vi "HitrapGUI.HTLE_TR6BT1.vi"() -> ()   [LabVIEW 2014, in "HitrapGUI.lvlib"]
uses:
  HitrapGUI.lvlib
  CSlibraries/GUILib/GUILib.userEventsMainType.ctl
  CSlibraries-extern/DimLVEvent/DimIndicators/DimIndicators.anyType.ctl
  CSlibraries/GUILib/GUILib.simpleNumeric.ctl
  CSlibraries/GUILib/GUILib.basicNumeric.ctl
  CSlibraries/UtilityLib/UtilityLib.valueStatus.ctl
  CSCore/CSSystem/CoreDefs/CoreDefs.rawDataType.ctl
  CSCore/CSSystem/CoreLib/CoreLib.double 2 byte array.vi
  CSlibraries/UtilityLib/UtilityLib.lvlib
  CSCore/CSSystem/CSSystemLib/CSSystemLib.lvlib
  CSlibraries-extern/DimLVEvent/DimIndicators/DimIndicators.lvlib
  CSCore/GUIs/GOGControllerGUI/GOGControllerGUI.lvlib
  CSlibraries/GUILib/GUILib.lvlib
  CSCore/CSSystem/CoreLib/CoreLib.lvlib
panel:
  in  "userEventsMain 2":T1
  in  "userEventsMain":T1
  in  "Next":bool
  in  "Previous":bool
  in  "APS_ch1":bool=TRUE
  in  "APS_ch1Ctl":T2 {"nom" step=1.0}
  in  "APS_ch2Ctl":T2 {"nom" step=1.0}
  in  "APS_ch2":bool=TRUE
  in  "All Low   All High":bool
  in  "High21":bool
  in  "High20":bool
  in  "High19":bool
  in  "High18":bool
  in  "High17":bool
  in  "High15":bool
  in  "High16":bool
  in  "High13":bool
  in  "High14":bool
  in  "High11":bool
  in  "High12":bool
  in  "High9":bool
  in  "High10":bool
  in  "High5":bool
  in  "High6":bool
  in  "High7":bool
  in  "High8":bool
  in  "High4":bool
  in  "High3":bool
  in  "High2":bool
  in  "High1":bool
  out "XY Graph":cluster{dbl, "Value":dbl}[](graph)
  in  "TR6BT1 SetModeCtl":T2 caption="TR6BT1Trap1Ctl" {"nom" step=1.0}
  in  "TR6BT1 SetMode":bool=TRUE
  in  "Enum":enum16{"Voltage1", "Voltage2"}(ring)
  in  "LowVoltage      HighVoltage":bool
  in  "TR6BT1Trap11Ctl":cluster{"nom":T3, "act":dbl, "inc":dbl} {"nom" step=1.0}
  in  "TR6BT1Trap10Ctl":cluster{"nom":T3, "act":dbl, "inc":dbl} {"nom" step=1.0}
  in  "TR6BT1Trap9Ctl":cluster{"nom":T3, "act":dbl, "inc":dbl} {"nom" step=1.0}
  in  "TR6BT1Trap7Ctl":cluster{"nom":T3, "act":dbl, "inc":dbl} {"nom" step=1.0}
  in  "TR6BT1Trap5Ctl":cluster{"nom":T3, "act":dbl, "inc":dbl} {"nom" step=1.0}
  in  "TR6BT1Trap12Ctl":cluster{"nom":T3, "act":dbl, "inc":dbl} {"nom" step=1.0}
  in  "TR6BT1Trap21Ctl":cluster{"nom":T3, "act":dbl, "inc":dbl} {"nom" step=1.0}
  in  "TR6BT1Trap8Ctl":cluster{"nom":T3, "act":dbl, "inc":dbl} {"nom" step=1.0}
  in  "TR6BT1Trap6Ctl":cluster{"nom":T3, "act":dbl, "inc":dbl} {"nom" step=1.0}
  in  "TR6BT1Trap4Ctl":cluster{"nom":T3, "act":dbl, "inc":dbl} {"nom" step=1.0}
  in  "TR6BT1Trap2Ctl":cluster{"nom":T3, "act":dbl, "inc":dbl} {"nom" step=1.0}
  in  "TR6BT1Trap3Ctl":cluster{"nom":T3, "act":dbl, "inc":dbl} {"nom" step=1.0}
  in  "TR6BT1Trap19Ctl":cluster{"nom":T3, "act":dbl, "inc":dbl} {"nom" step=1.0}
  in  "TR6BT1Trap20Ctl":cluster{"nom":T3, "act":dbl, "inc":dbl} {"nom" step=1.0}
  in  "TR6BT1Trap18Ctl":cluster{"nom":T3, "act":dbl, "inc":dbl} {"nom" step=1.0}
  in  "TR6BT1Trap17Ctl":cluster{"nom":T3, "act":dbl, "inc":dbl} {"nom" step=1.0}
  in  "TR6BT1Trap16Ctl":cluster{"nom":T3, "act":dbl, "inc":dbl} {"nom" step=1.0}
  in  "TR6BT1Trap15Ctl":cluster{"nom":T3, "act":dbl, "inc":dbl} {"nom" step=1.0}
  in  "TR6BT1Trap14Ctl":cluster{"nom":T3, "act":dbl, "inc":dbl} {"nom" step=1.0}
  in  "TR6BT1Trap13Ctl":cluster{"nom":T3, "act":dbl, "inc":dbl} {"nom" step=1.0}
  in  "TR6BT1Trap1Ctl":cluster{"nom":T3, "act":dbl, "inc":dbl} {"nom" step=1.0}
  in  "TR6BT1Trap11_HCtl":cluster{"nom":T3, "act":dbl, "inc":dbl} {"nom" step=1.0}
  in  "TR6BT1Trap10_HCtl":cluster{"nom":T3, "act":dbl, "inc":dbl} {"nom" step=1.0}
  in  "TR6BT1Trap4_HCtl":cluster{"nom":T3, "act":dbl, "inc":dbl} {"nom" step=1.0}
  in  "TR6BT1Trap9_HCtl":cluster{"nom":T3, "act":dbl, "inc":dbl} {"nom" step=1.0}
  in  "TR6BT1Trap12_HCtl":cluster{"nom":T3, "act":dbl, "inc":dbl} {"nom" step=1.0}
  in  "TR6BT1Trap21_HCtl":cluster{"nom":T3, "act":dbl, "inc":dbl} {"nom" step=1.0}
  in  "TR6BT1Trap8_HCtl":cluster{"nom":T3, "act":dbl, "inc":dbl} {"nom" step=1.0}
  in  "TR6BT1Trap7_HCtl":cluster{"nom":T3, "act":dbl, "inc":dbl} {"nom" step=1.0}
  in  "TR6BT1Trap6_HCtl":cluster{"nom":T3, "act":dbl, "inc":dbl} {"nom" step=1.0}
  in  "TR6BT1Trap5_HCtl":cluster{"nom":T3, "act":dbl, "inc":dbl} {"nom" step=1.0}
  in  "TR6BT1Trap3_HCtl":cluster{"nom":T3, "act":dbl, "inc":dbl} {"nom" step=1.0}
  in  "TR6BT1Trap2_HCtl":cluster{"nom":T3, "act":dbl, "inc":dbl} {"nom" step=1.0}
  in  "TR6BT1Trap20_HCtl":cluster{"nom":T3, "act":dbl, "inc":dbl} {"nom" step=1.0}
  in  "TR6BT1Trap17_HCtl":cluster{"nom":T3, "act":dbl, "inc":dbl} {"nom" step=1.0}
  in  "TR6BT1Trap18_HCtl":cluster{"nom":T3, "act":dbl, "inc":dbl} {"nom" step=1.0}
  in  "TR6BT1Trap19_HCtl":cluster{"nom":T3, "act":dbl, "inc":dbl} {"nom" step=1.0}
  in  "TR6BT1Trap16_HCtl":cluster{"nom":T3, "act":dbl, "inc":dbl} {"nom" step=1.0}
  in  "TR6BT1Trap15_HCtl":cluster{"nom":T3, "act":dbl, "inc":dbl} {"nom" step=1.0}
  in  "TR6BT1Trap14_HCtl":cluster{"nom":T3, "act":dbl, "inc":dbl} {"nom" step=1.0}
  in  "TR6BT1Trap13_HCtl":cluster{"nom":T3, "act":dbl, "inc":dbl} {"nom" step=1.0}
  in  "TR6BT1Trap1_HCtl":cluster{"nom":T3, "act":dbl, "inc":dbl} {"nom" step=1.0}
  in  "TR6BT1Trap2":bool=TRUE
  in  "TR6BT1Trap21":bool=TRUE
  in  "TR6BT1Trap20":bool=TRUE
  in  "TR6BT1Trap19":bool=TRUE
  in  "TR6BT1Trap18":bool=TRUE
  in  "TR6BT1Trap17":bool=TRUE
  in  "TR6BT1Trap16":bool=TRUE
  in  "TR6BT1Trap15":bool=TRUE
  in  "TR6BT1Trap14":bool=TRUE
  in  "TR6BT1Trap13":bool=TRUE
  in  "TR6BT1Trap12":bool=TRUE
  in  "TR6BT1Trap11":bool=TRUE
  in  "TR6BT1Trap10":bool=TRUE
  in  "TR6BT1Trap9":bool=TRUE
  in  "TR6BT1Trap8":bool=TRUE
  in  "TR6BT1Trap7":bool=TRUE
  in  "TR6BT1Trap6":bool=TRUE
  in  "TR6BT1Trap5":bool=TRUE
  in  "TR6BT1Trap4":bool=TRUE
  in  "TR6BT1Trap3":bool=TRUE
  in  "TR6BT1Trap1":bool=TRUE
  in  "TR6BT1Trap12/2":bool=TRUE
  in  "TR6BT1Trap11/8":bool=TRUE
  in  "TR6BT1Trap11/7":bool=TRUE
  in  "TR6BT1Trap11/6":bool=TRUE
  in  "TR6BT1Trap11/5":bool=TRUE
  in  "TR6BT1Trap11/4":bool=TRUE
  in  "TR6BT1Trap11/3":bool=TRUE
  in  "TR6BT1Trap11/2":bool=TRUE
  in  "TR6BT1Trap10/2":bool=TRUE
  in  "TR6BT1Trap12/2_H":bool=TRUE
  in  "TR6BT1Trap11/8_H":bool=TRUE
  in  "TR6BT1Trap11/7_H":bool=TRUE
  in  "TR6BT1Trap11/6_H":bool=TRUE
  in  "TR6BT1Trap11/5_H":bool=TRUE
  in  "TR6BT1Trap11/4_H":bool=TRUE
  in  "TR6BT1Trap11/3_H":bool=TRUE
  in  "TR6BT1Trap11/2_H":bool=TRUE
  in  "TR6BT1Trap10/2_H":bool=TRUE
  in  "TR6BT1Trap12/2Ctl":T2 {"nom" step=1.0}
  in  "TR6BT1Trap11/8Ctl":T2 {"nom" step=1.0}
  in  "TR6BT1Trap11/7Ctl":T2 {"nom" step=1.0}
  in  "TR6BT1Trap11/6Ctl":T2 {"nom" step=1.0}
  in  "TR6BT1Trap11/5Ctl":T2 {"nom" step=1.0}
  in  "TR6BT1Trap11/4Ctl":T2 {"nom" step=1.0}
  in  "TR6BT1Trap11/3Ctl":T2 {"nom" step=1.0}
  in  "TR6BT1Trap11/2Ctl":T2 {"nom" step=1.0}
  in  "TR6BT1Trap10/2Ctl":T2 {"nom" step=1.0}
  in  "TR6BT1Trap12/2_HCtl":T2 {"nom" step=1.0}
  in  "TR6BT1Trap11/8_HCtl":T2 {"nom" step=1.0}
  in  "TR6BT1Trap11/7_HCtl":T2 {"nom" step=1.0}
  in  "TR6BT1Trap11/6_HCtl":T2 {"nom" step=1.0}
  in  "TR6BT1Trap11/5_HCtl":T2 {"nom" step=1.0}
  in  "TR6BT1Trap11/4_HCtl":T2 {"nom" step=1.0}
  in  "TR6BT1Trap11/3_HCtl":T2 {"nom" step=1.0}
  in  "TR6BT1Trap11/2_HCtl":T2 {"nom" step=1.0}
  in  "TR6BT1Trap10/2_HCtl":T2 {"nom" step=1.0}
  in  "TR6BT1Trap17_H":bool=TRUE
  in  "TR6BT1Trap16_H":bool=TRUE
  in  "TR6BT1Trap15_H":bool=TRUE
  in  "TR6BT1Trap14_H":bool=TRUE
  in  "TR6BT1Trap13_H":bool=TRUE
  in  "TR6BT1Trap12_H":bool=TRUE
  in  "TR6BT1Trap8_H":bool=TRUE
  in  "TR6BT1Trap7_H":bool=TRUE
  in  "TR6BT1Trap5_H":bool=TRUE
  in  "TR6BT1Trap4_H":bool=TRUE
  in  "TR6BT1Trap3_H":bool=TRUE
  in  "TR6BT1Trap2_H":bool=TRUE
  in  "TR6BT1Trap21_H":bool=TRUE
  in  "TR6BT1Trap20_H":bool=TRUE
  in  "TR6BT1Trap19_H":bool=TRUE
  in  "TR6BT1Trap18_H":bool=TRUE
  in  "TR6BT1Trap11_H":bool=TRUE
  in  "TR6BT1Trap10_H":bool=TRUE
  in  "TR6BT1Trap9_H":bool=TRUE
  in  "TR6BT1Trap6_H":bool=TRUE
  in  "TR6BT1Trap1_H":bool=TRUE
  in  "OK Button":bool
  in  "analog1Ctl":T2 {"nom" step=1.0}
  in  "analog1":bool=TRUE
  out "subSystem1State":string
  in  "subSystem1":bool
  out "subSystem1StateQuality":string
  in  "subControllersIgnoredDIM":T4
  in  "iniData":string
  in  "stop":bool
  in  "dummy":bool
  in  "parentSystem":bool
  in  "userEvent":refnum<user-event>
  # "TR6BT1"
  # "Amplifier"
  # "1"
  # "2"
  # "3"
  # "4"
  # "5"
  # "6"
  # "7"
  # "8"
  # "9"
  # "10"
  # "11"
  # "12"
  # "13"
  # "14"
  # "15"
  # "16"
  # "17"
  # "18"
  # "19"
  # "20"
  # "21"
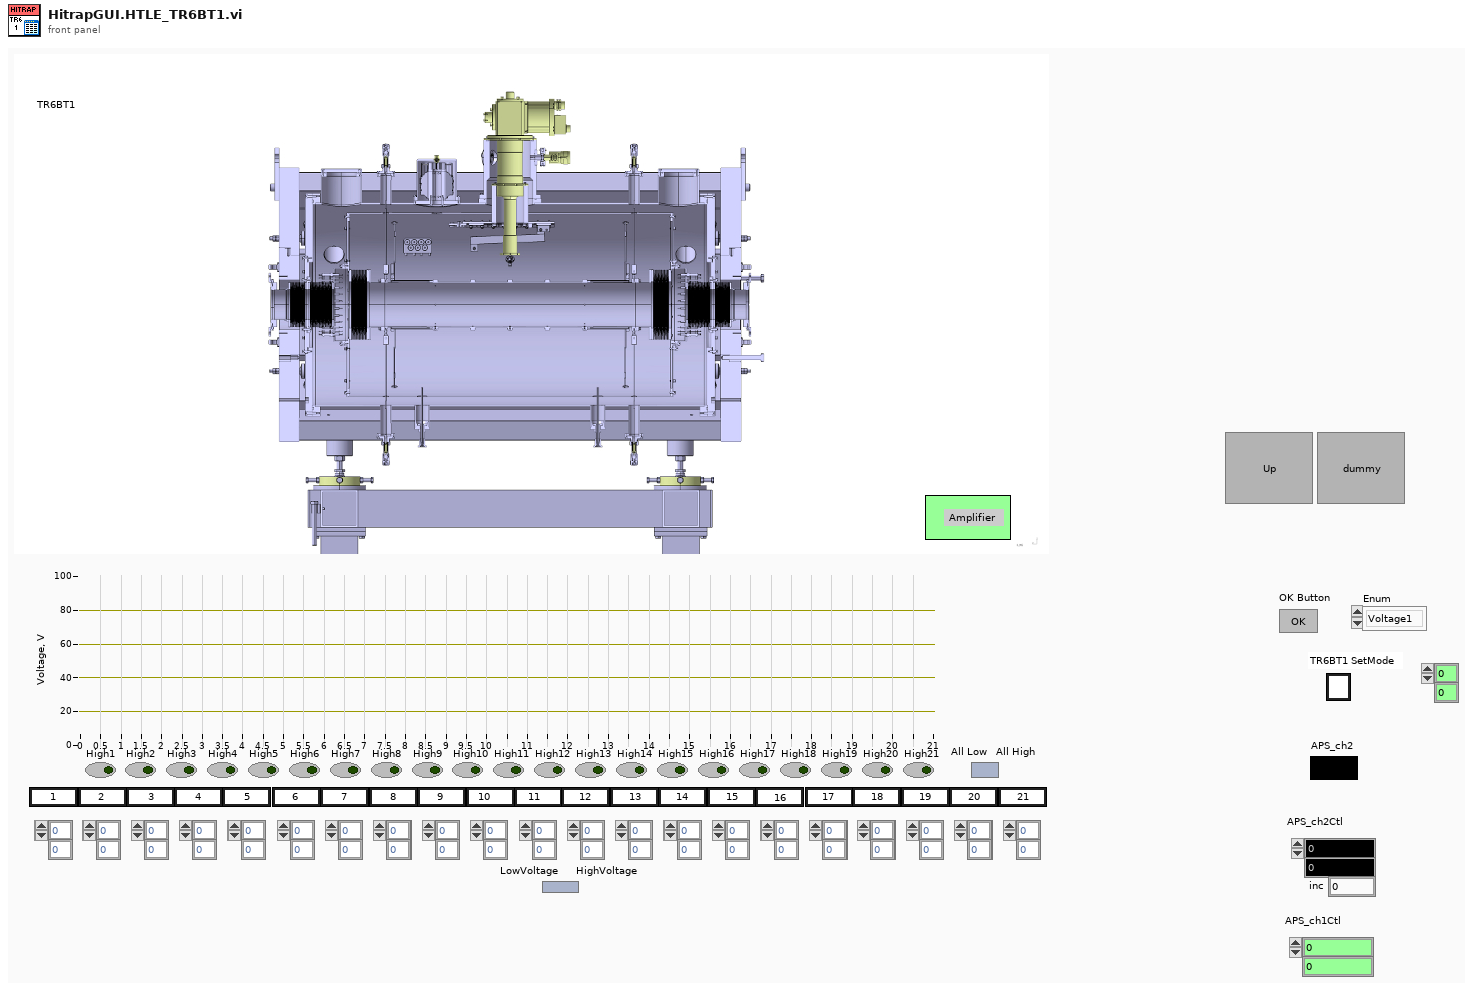
[diagram p1: front panel]
types:
  T1 = typedef "GUILib.lvlib/GUILib.userEventsMainType.ctl" = cluster{"data":string, "dataType":i32}
  T2 = typedef "GUILib.lvlib/GUILib.simpleNumeric.ctl" = cluster{"nom":T3, "act":dbl, "inc":dbl}
  T3 = typedef "GUILib.lvlib/GUILib.basicNumeric.ctl" = dbl
  T4 = typedef "DimIndicators.lvlib/DimIndicators.anyType.ctl" = cluster{"data":string, "no link":bool, "quality":i32, "timeStamp":dbl}
  T5 = typedef "UtilityLib.lvlib/UtilityLib.valueStatus.ctl" = enum16{"no info available", "stand by/off", "on", "warning", "alarm/malfunction", "not implemented", "user action required", "important information", "system default", "control default", "indicator default", "button default"}
  T6 = typedef "CoreDefs.rawDataType.ctl" = i8[]
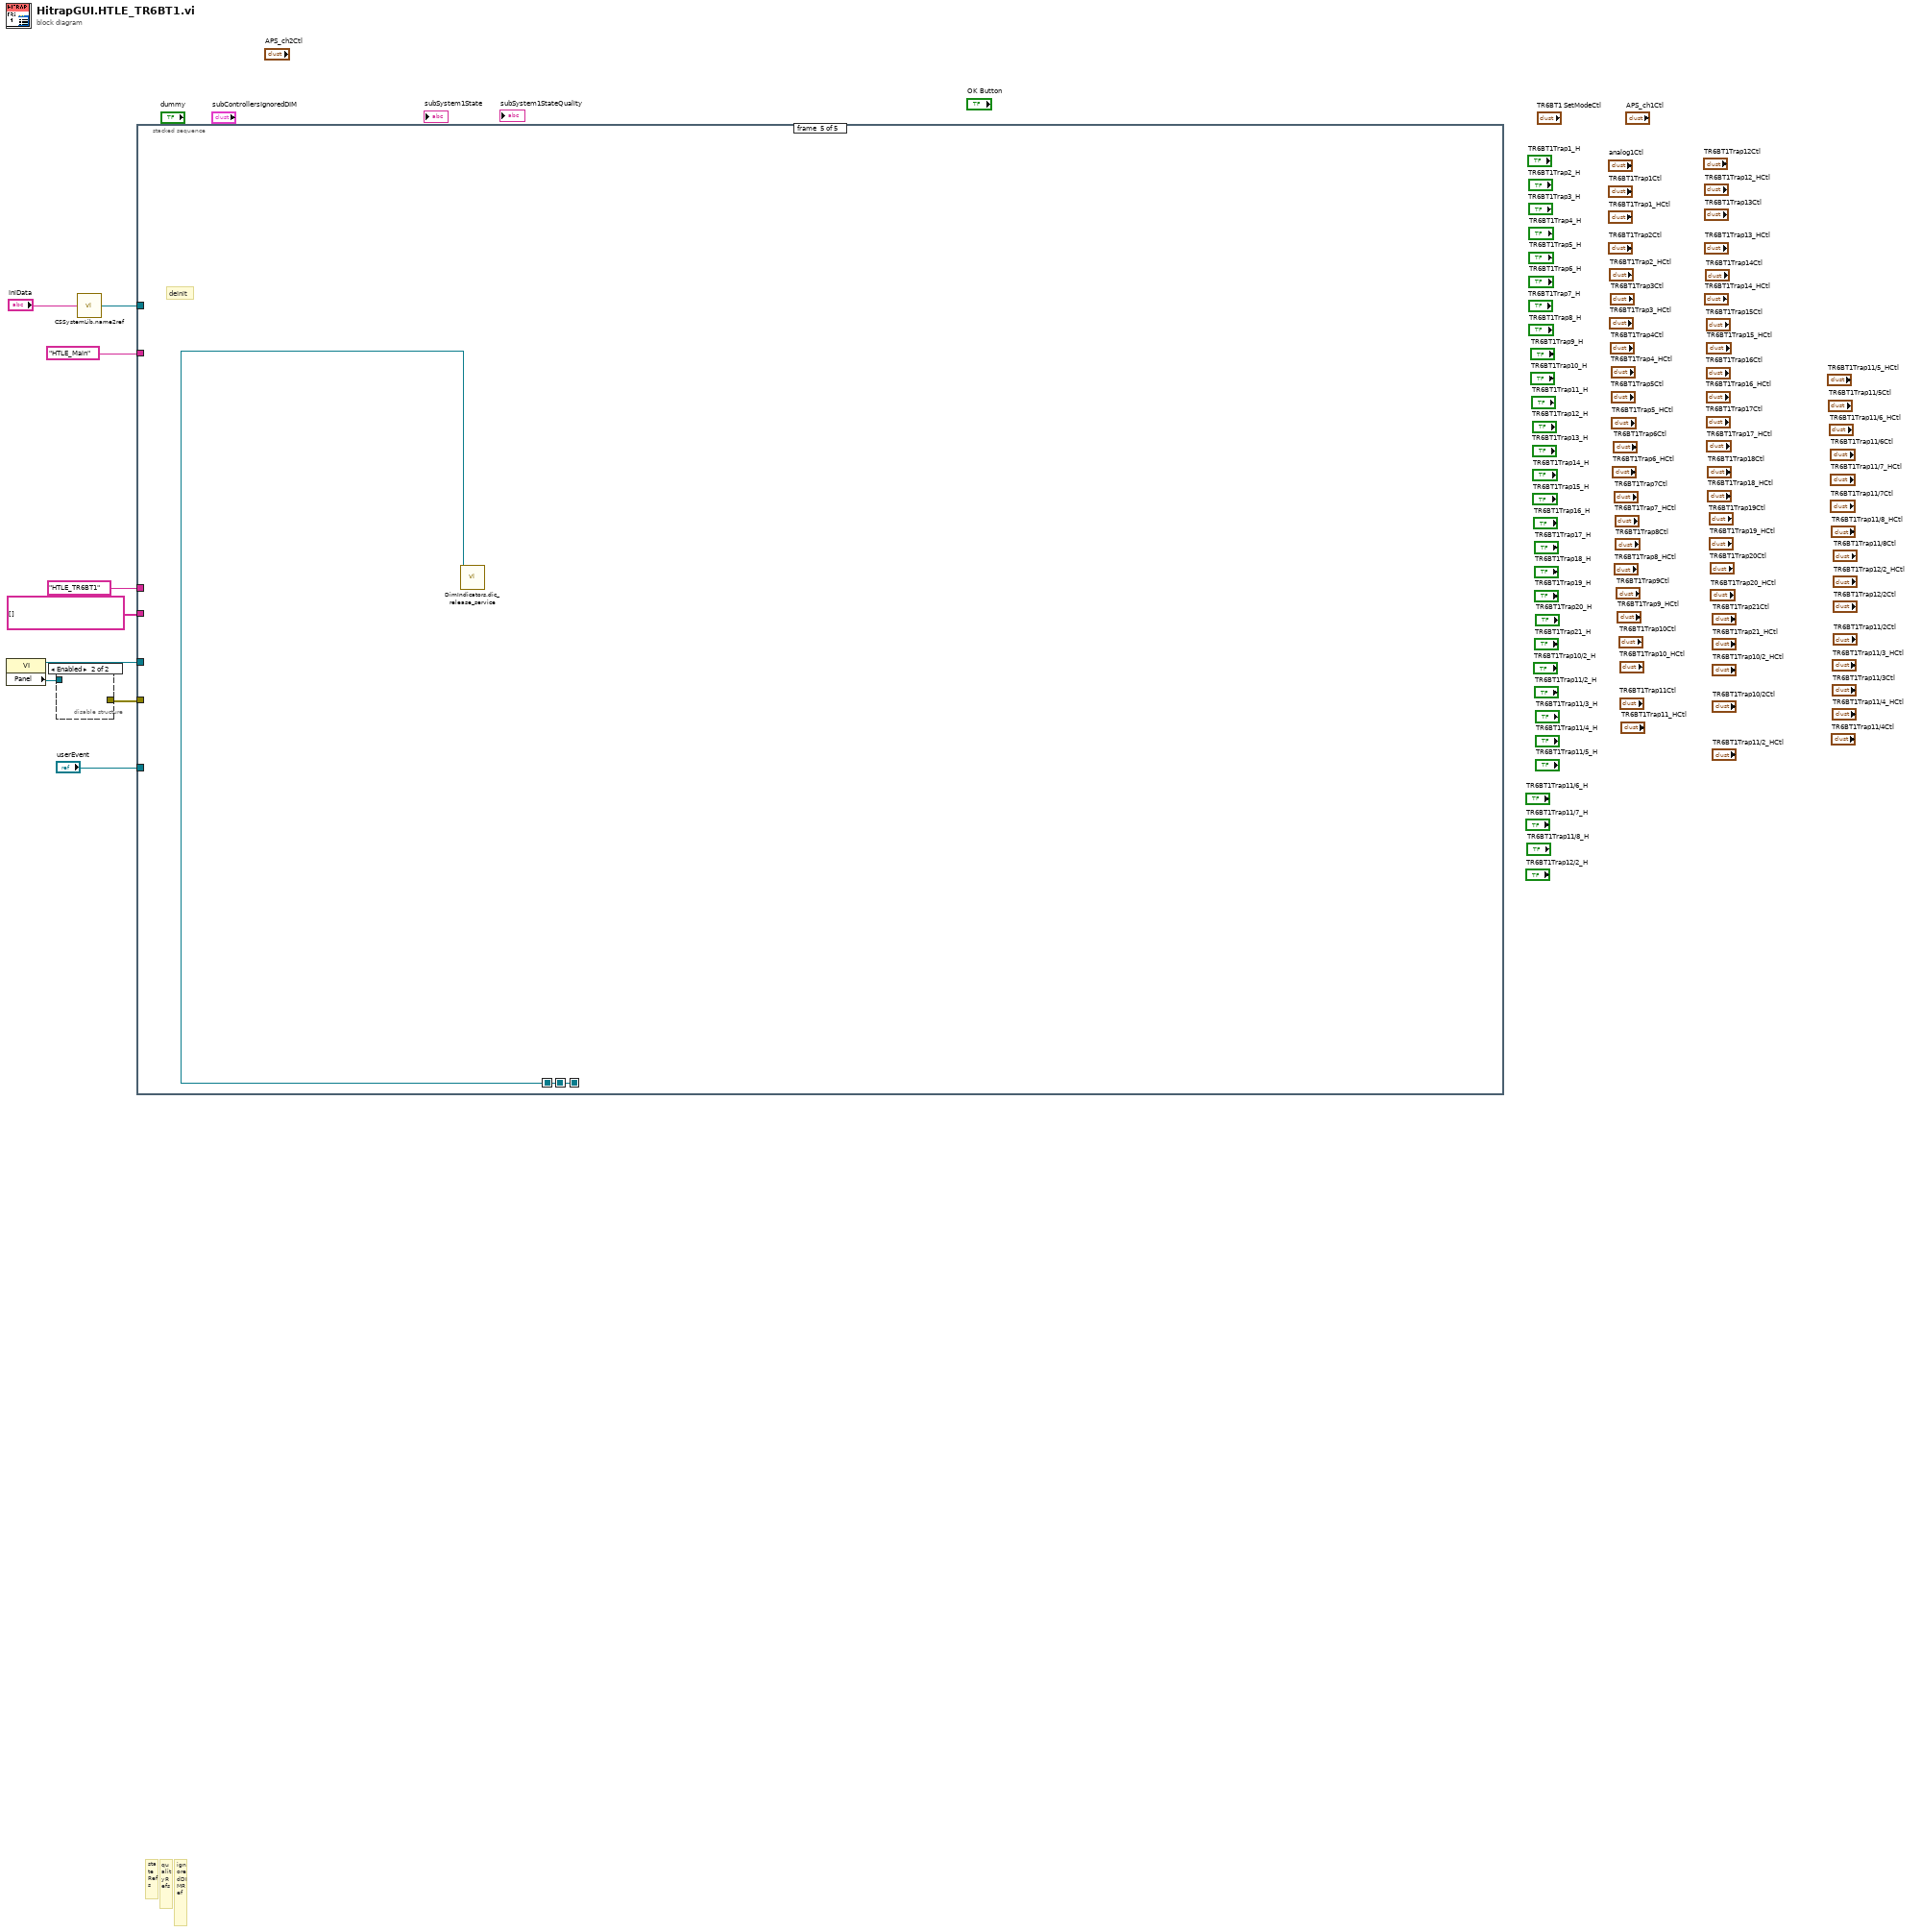
[diagram p0: block diagram]
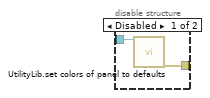
[diagram p2: hidden frame]
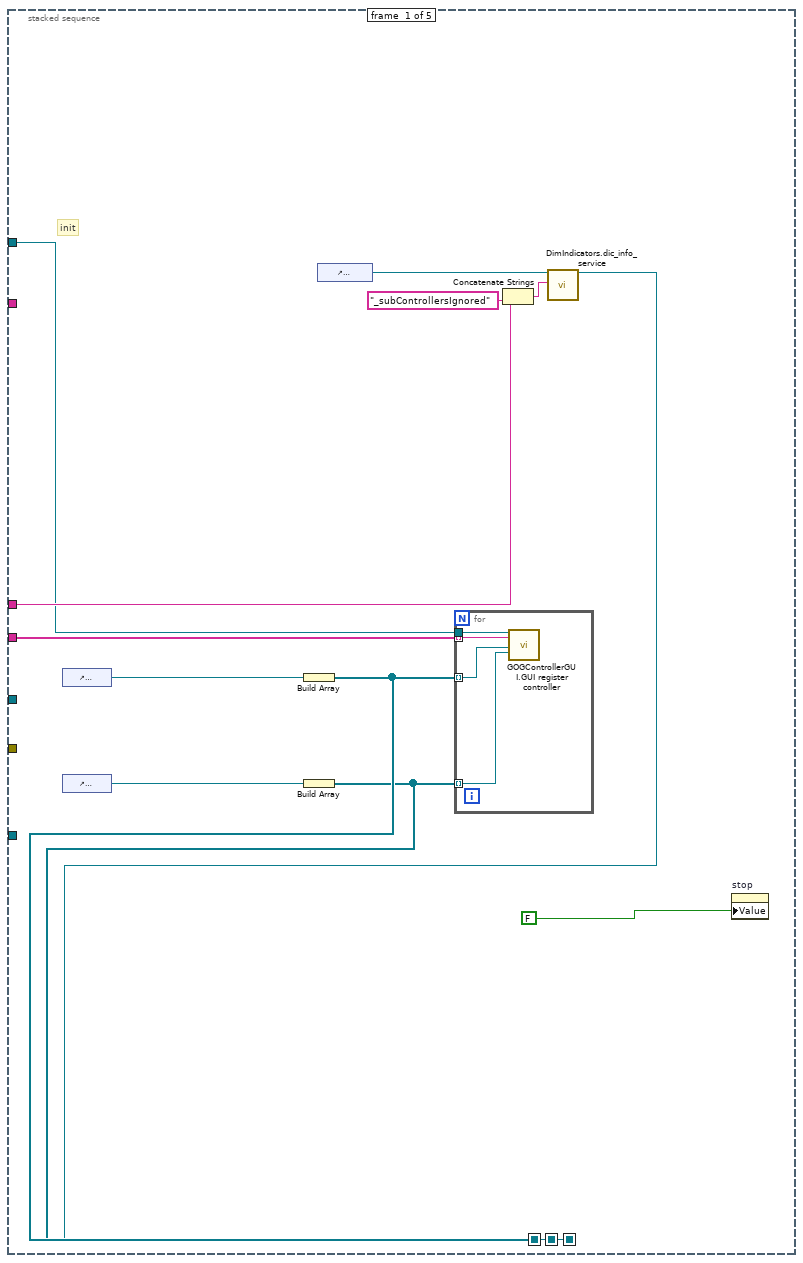
[diagram p3: hidden frame]
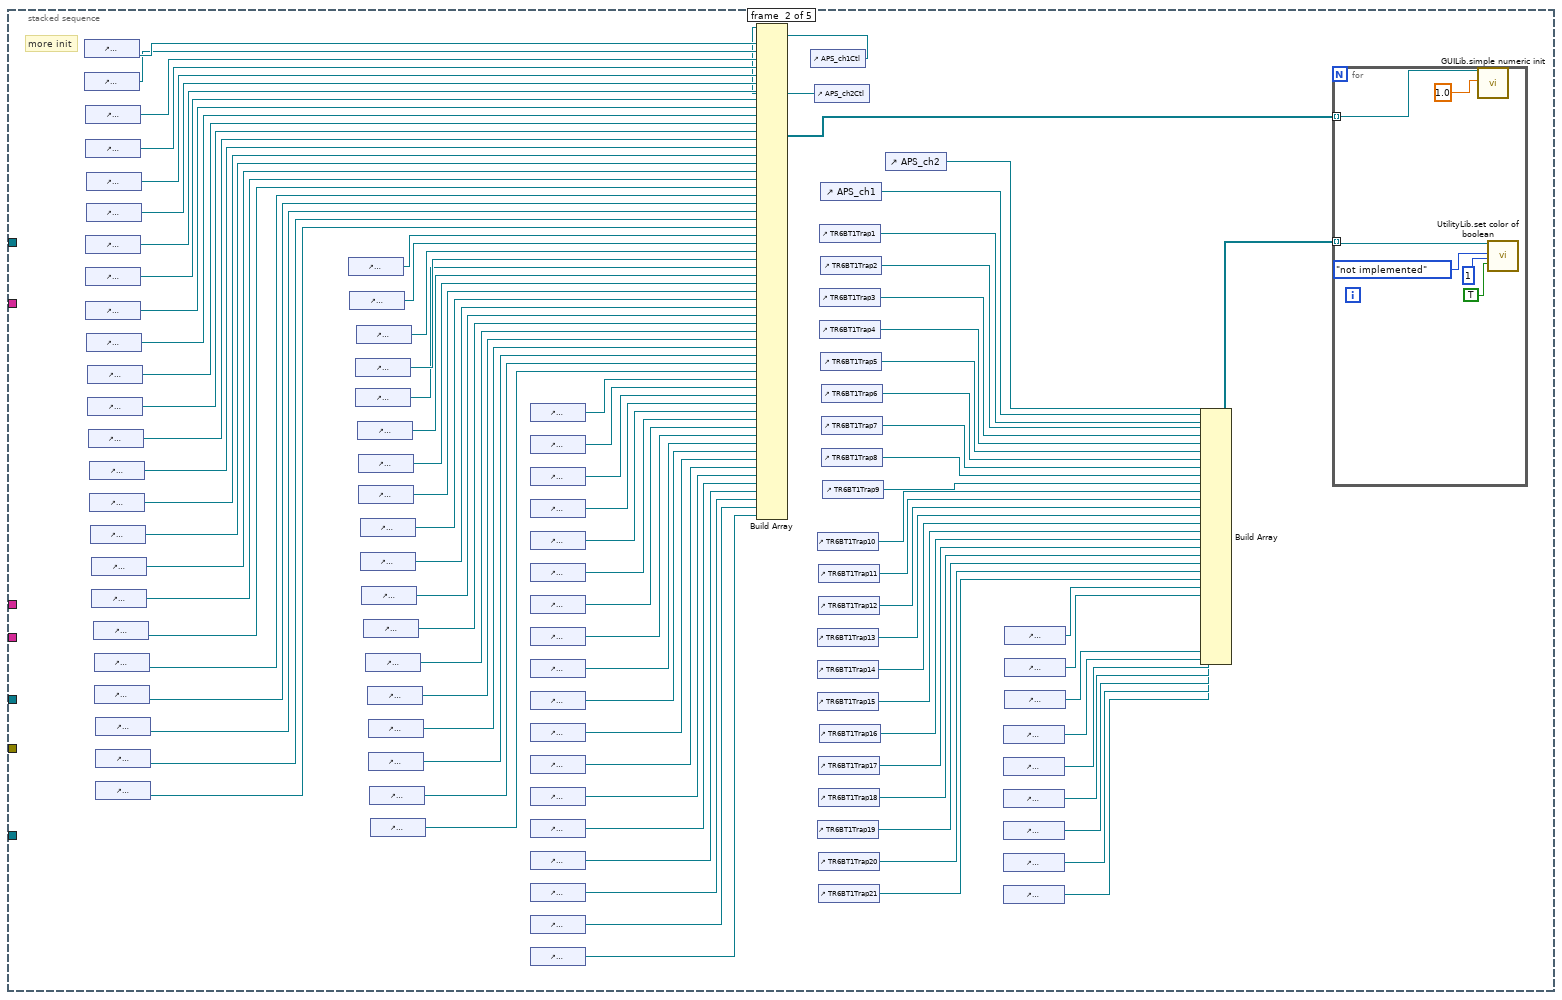
[diagram p4: hidden frame]
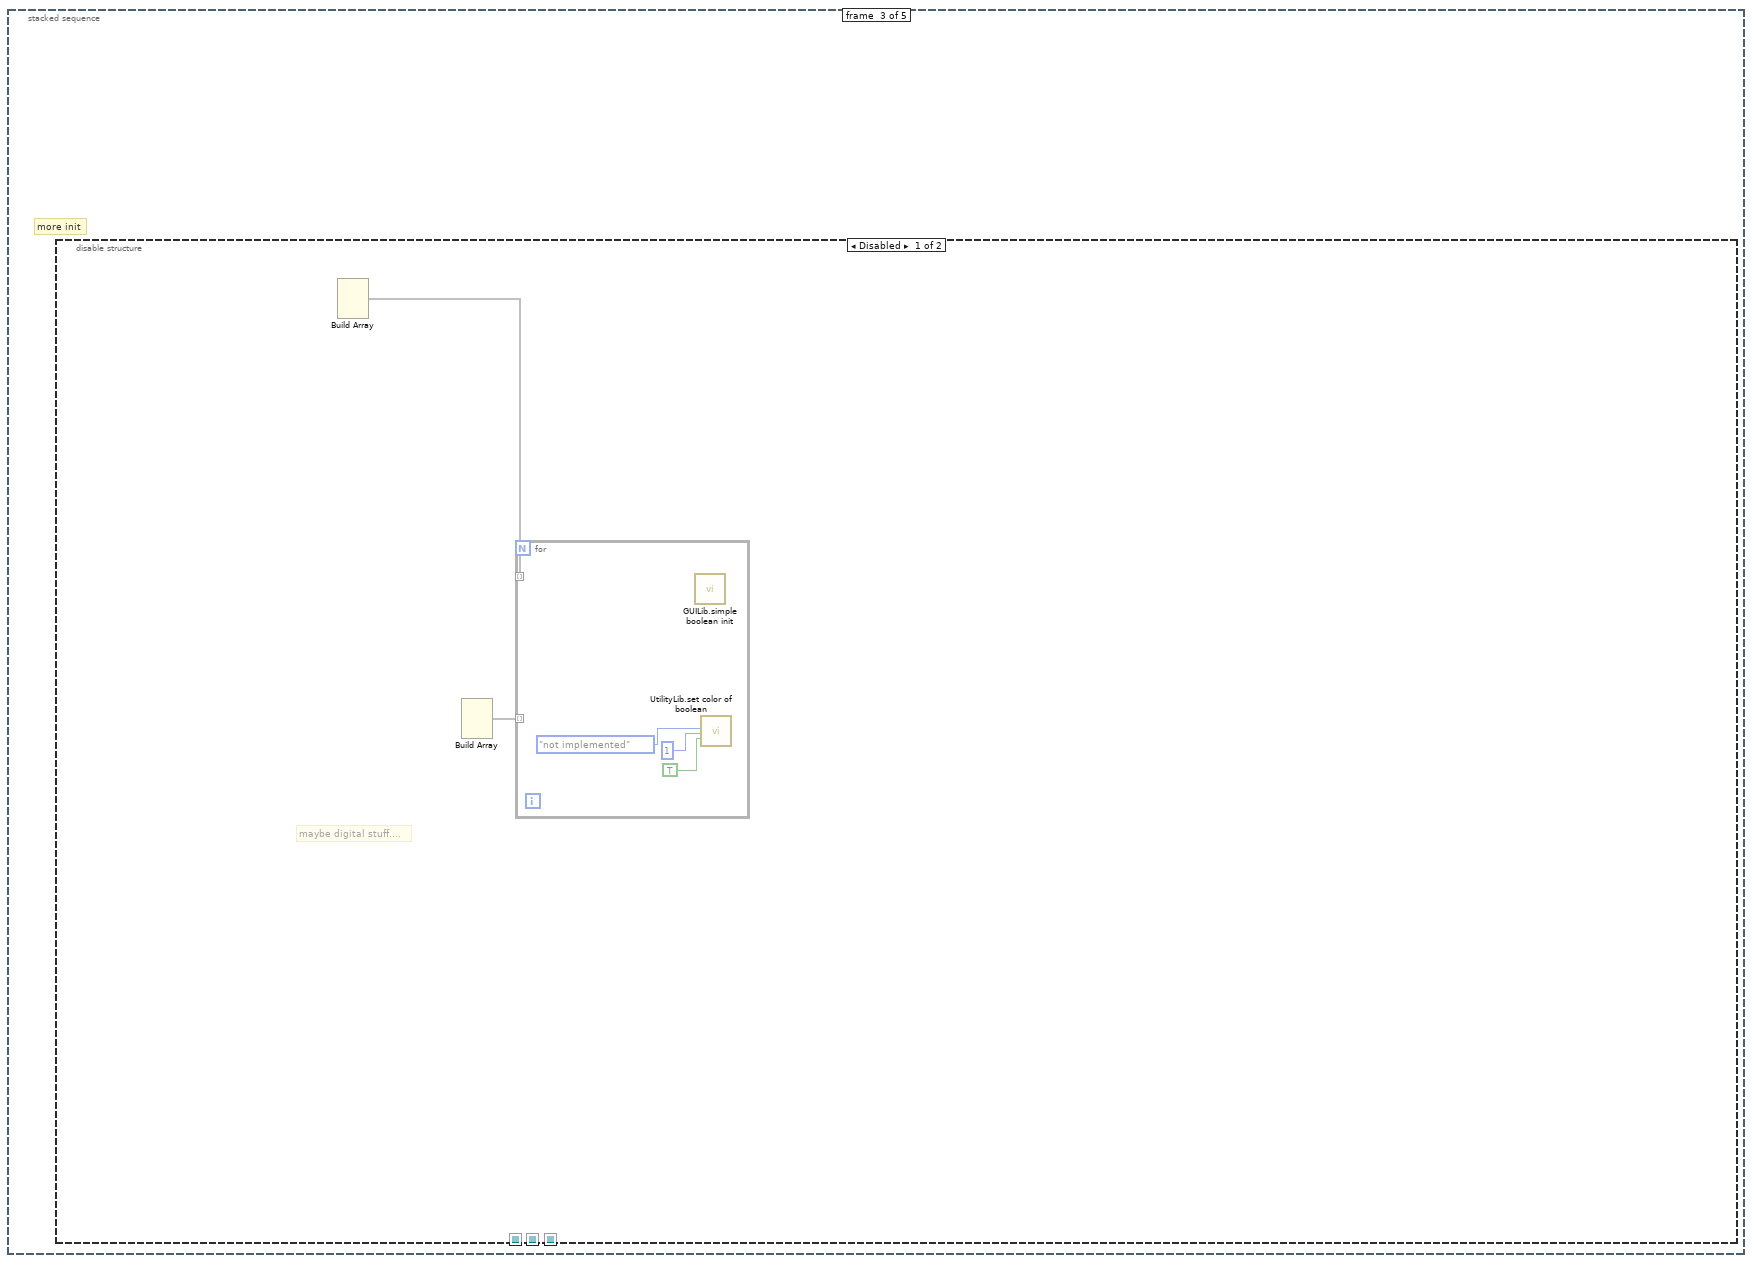
[diagram p5: hidden frame]
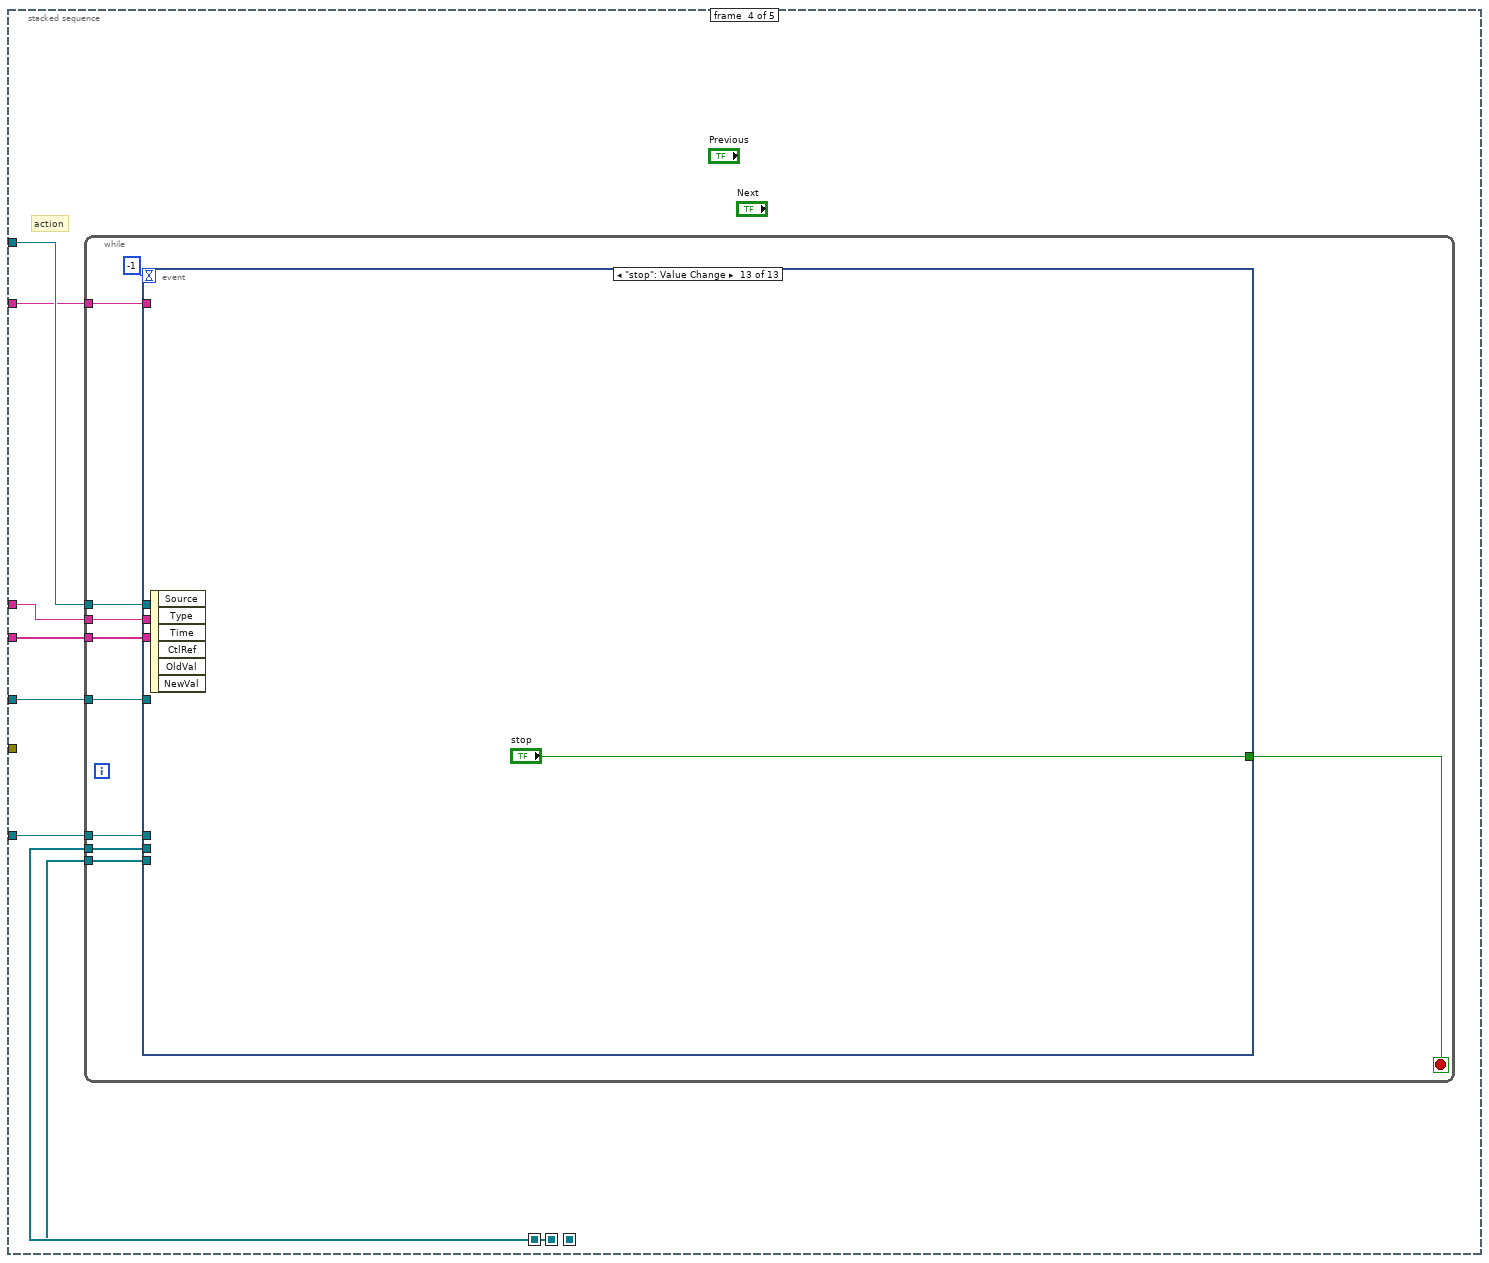
[diagram p7: hidden frame]
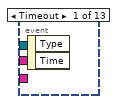
[diagram p8: hidden frame]
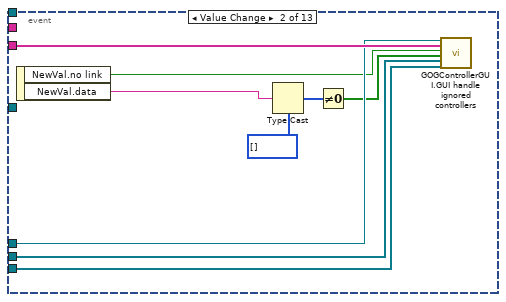
[diagram p9: hidden frame]
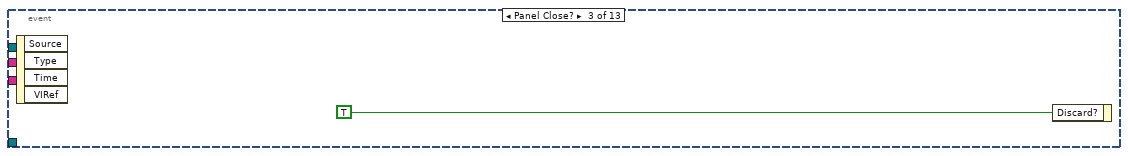
[diagram p10: hidden frame]
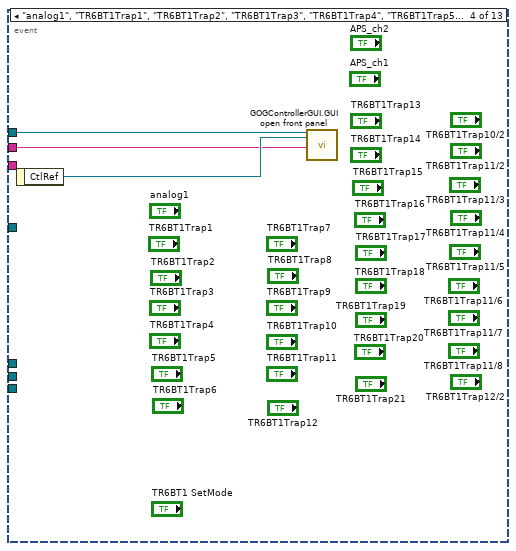
[diagram p11: hidden frame]
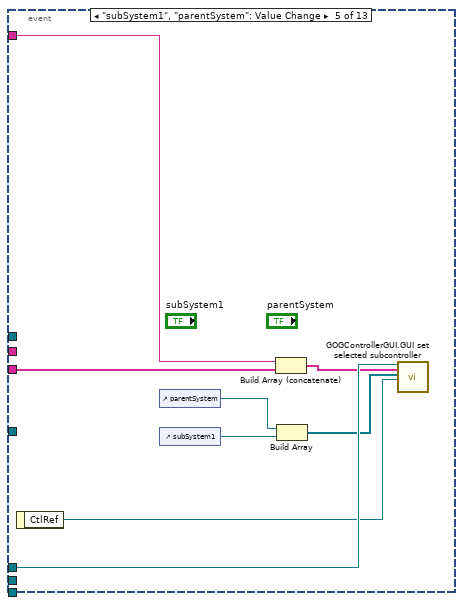
[diagram p12: hidden frame]
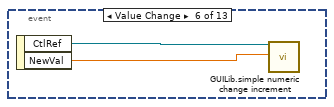
[diagram p13: hidden frame]
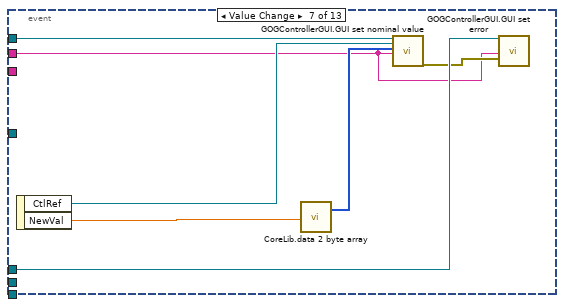
[diagram p14: hidden frame]
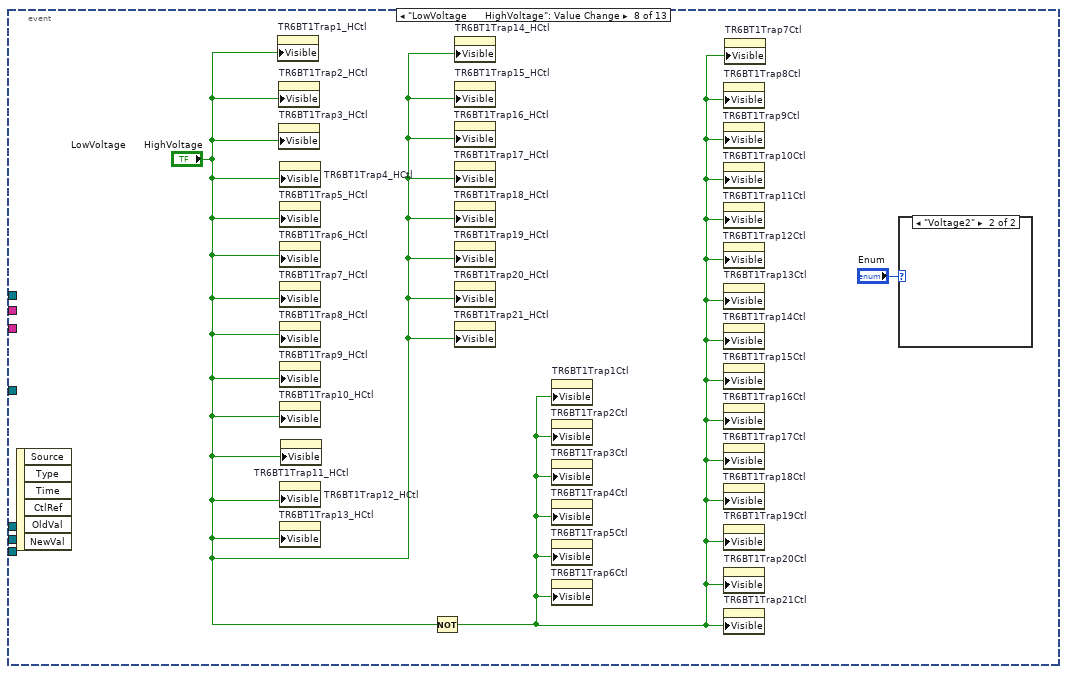
[diagram p15: hidden frame]
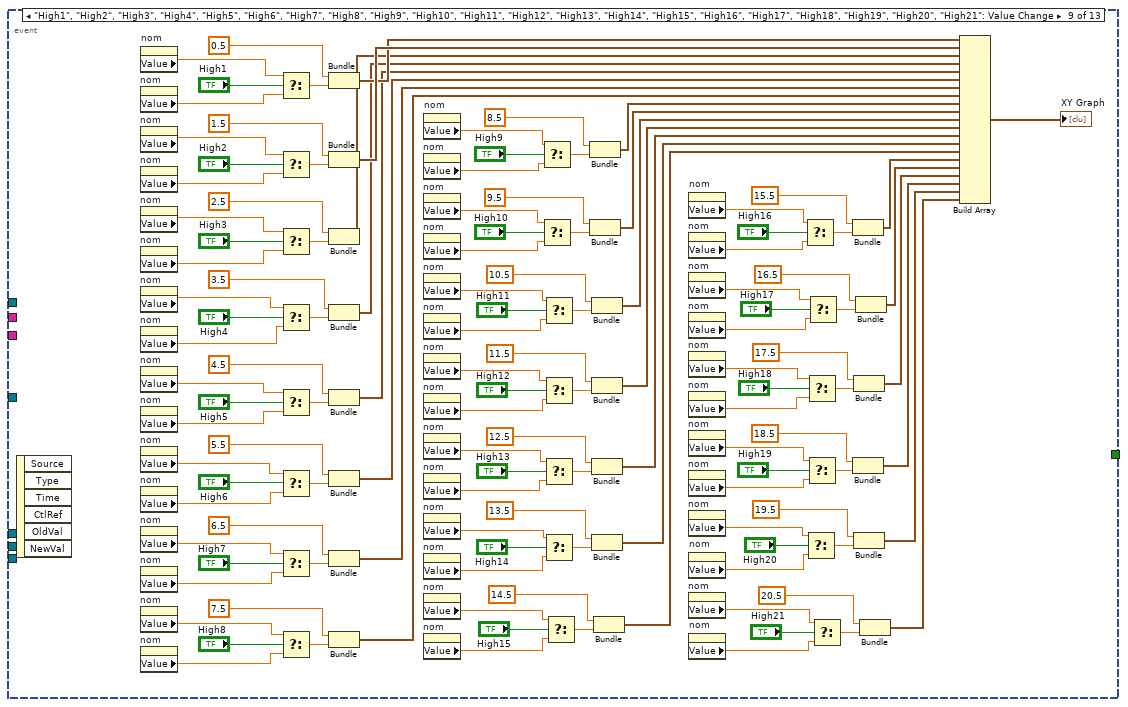
[diagram p17: hidden frame]
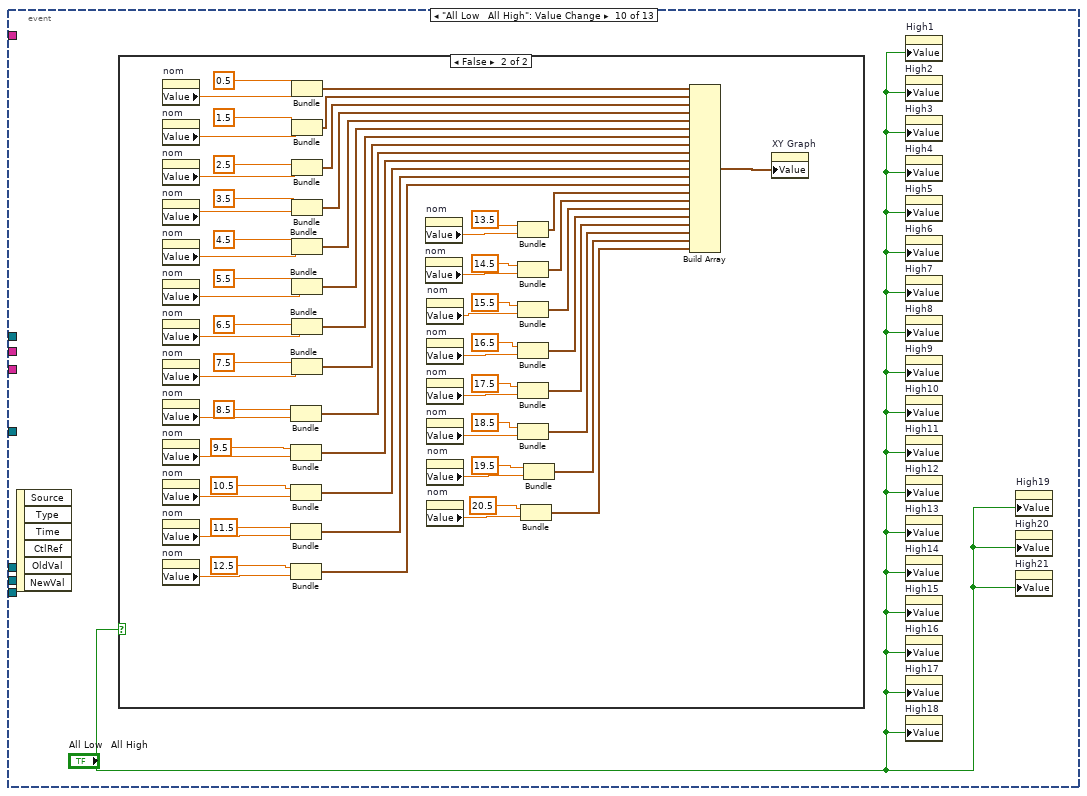
[diagram p18: hidden frame]
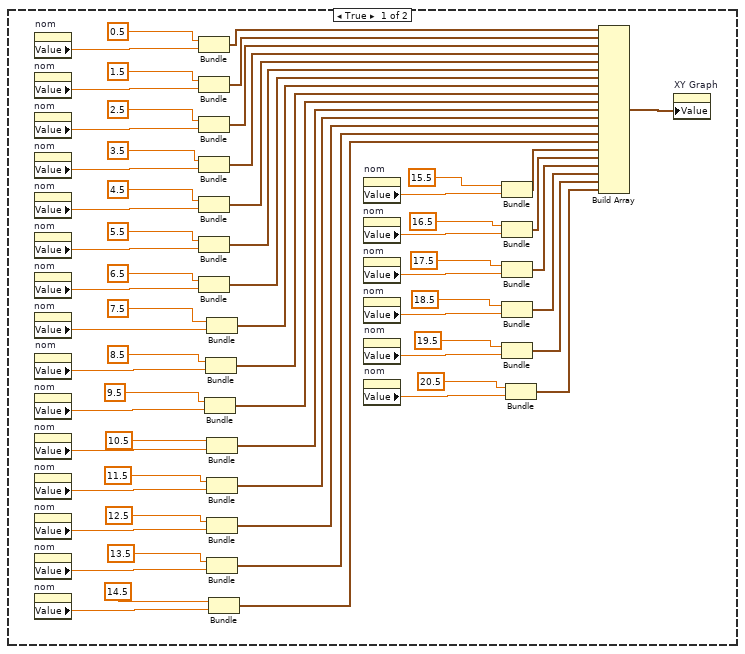
[diagram p19: hidden frame]
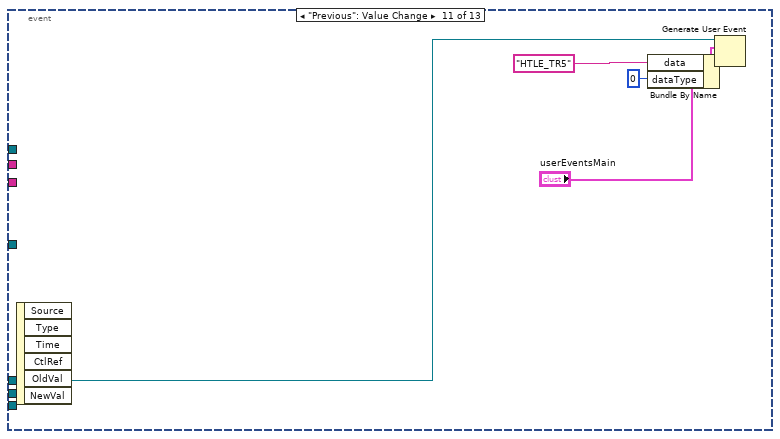
[diagram p20: hidden frame]
diagram:
  # "qualityRefs"
  # "ignoredDIMRef"
  # "stateRefs"
  n1 = property class="VI"() -> (reference out=w7:refnum<vi>, "Panel"=w8:refnum<vi>)  [unwired: 2 in, 1 out]
  n2 = disable-structure shown="Enabled" {
    disable-tunnel: w8 -> [w11 _]
    disable-tunnel: [w10 _] -> w6
    frame Disabled {
      n3 = call "UtilityLib.set colors of panel to defaults.vi"("Front Panel"=w11) -> ("error out"=w10:errorcluster)  [unwired: 18 in]
    }
    frame Enabled {
    }
  }
  n4 = call "CSSystemLib.name2ref.vi"("name"="iniData") -> ("obj refnum"=w2:refnum<vi>)
  n5 = stacked-sequence {
    seq-local: [w13 _ _ _ _] -> [_ _ _ _ w453]
    seq-local: [w14 _ _ _ _] -> [_ _ _ w139 _]
    seq-local: [w12 _ _ _ _] -> [_ _ _ w138 _]
    tunnel: "userEvent" -> [_ _ _ w142 _]
    tunnel: w7 -> [_ _ _ w141 _]
    tunnel: w6 -> [_ _ _ _ _]
    tunnel: "HTLE_TR6BT1" -> [w19 _ _ w136 _]
    tunnel: string[] [] -> [w18 _ _ w140 _]
    tunnel: w2 -> [w17 _ _ w137 _]
    tunnel: "HTLE_Main" -> [_ _ _ w135 _]
    frame #0 {
      # "init"
      n6 = control-ref of="dummySubSystemState"() -> (w16:refnum<vi>)
      n7 = control-ref of="dummySubSystemStateQuality"() -> (w15:refnum<vi>)
      n8 = Build Array(w16) -> (w14:refnum<vi>[])
      n9 = Build Array(w15) -> (w12:refnum<vi>[])
      n10 = control-ref of="subControllersIgnoredDIM"() -> (w20:refnum<vi>)
      n11 = for {
        tunnel: w14 -> [w27] mode=indexing
        tunnel: w18 -> [w25] mode=indexing
        tunnel: w12 -> [w24] mode=indexing
        tunnel: w17 -> [w26]
        n12 = call "GOGControllerGUI.GUI register controller.vi"("i ref in"=w26, "controllerName"=w25, "subSystemState"=w27, "subSystemStateQuality"=w24) -> ()  [unwired: 14 in, 2 out]
      }
      n13 = Concatenate Strings(w19, "_subControllersIgnored" ("string")) -> (w22:string)
      n14 = call "DimIndicators.dic_info_service.vi"("controlRef"=w20, "serviceName"=w22) -> ("controlRef out"=w13:refnum<vi>)  [unwired: 16 in, 1 out]
      n15 = property on="stop" class="Bool (strict)"("Value"=FALSE ("stop")) -> ()  [unwired: 2 in, 2 out]
    }
    frame #1 {
      # "more init"
      n16 = control-ref of="TR6BT1Trap1Ctl"() -> (w123:refnum<vi>)
      n17 = control-ref of="TR6BT1Trap1_HCtl"() -> (w119:refnum<vi>)
      n18 = control-ref of="TR6BT1Trap2Ctl"() -> (w118:refnum<vi>)
      n19 = control-ref of="TR6BT1Trap2_HCtl"() -> (w117:refnum<vi>)
      n20 = control-ref of="TR6BT1Trap4Ctl"() -> (w114:refnum<vi>)
      n21 = control-ref of="TR6BT1Trap4_HCtl"() -> (w113:refnum<vi>)
      n22 = control-ref of="TR6BT1Trap5Ctl"() -> (w112:refnum<vi>)
      n23 = control-ref of="TR6BT1Trap3Ctl"() -> (w116:refnum<vi>)
      n24 = control-ref of="TR6BT1Trap3_HCtl"() -> (w115:refnum<vi>)
      n25 = control-ref of="TR6BT1Trap5_HCtl"() -> (w111:refnum<vi>)
      n26 = control-ref of="TR6BT1Trap6Ctl"() -> (w110:refnum<vi>)
      n27 = control-ref of="TR6BT1Trap6_HCtl"() -> (w109:refnum<vi>)
      n28 = control-ref of="TR6BT1Trap7Ctl"() -> (w108:refnum<vi>)
      n29 = control-ref of="TR6BT1Trap7_HCtl"() -> (w107:refnum<vi>)
      n30 = control-ref of="TR6BT1Trap8Ctl"() -> (w106:refnum<vi>)
      n31 = control-ref of="TR6BT1Trap8_HCtl"() -> (w105:refnum<vi>)
      n32 = control-ref of="TR6BT1Trap9Ctl"() -> (w104:refnum<vi>)
      n33 = control-ref of="TR6BT1Trap9_HCtl"() -> (w103:refnum<vi>)
      n34 = control-ref of="TR6BT1Trap10Ctl"() -> (w101:refnum<vi>)
      n35 = control-ref of="TR6BT1Trap10_HCtl"() -> (w100:refnum<vi>)
      n36 = control-ref of="TR6BT1Trap11Ctl"() -> (w99:refnum<vi>)
      n37 = control-ref of="TR6BT1Trap11_HCtl"() -> (w98:refnum<vi>)
      n38 = control-ref of="TR6BT1Trap12Ctl"() -> (w97:refnum<vi>)
      n39 = control-ref of="TR6BT1Trap12_HCtl"() -> (w96:refnum<vi>)
      n40 = control-ref of="TR6BT1Trap13Ctl"() -> (w95:refnum<vi>)
      n41 = control-ref of="TR6BT1Trap13_HCtl"() -> (w94:refnum<vi>)
      n42 = control-ref of="TR6BT1Trap14_HCtl"() -> (w92:refnum<vi>)
      n43 = control-ref of="TR6BT1Trap15Ctl"() -> (w91:refnum<vi>)
      n44 = control-ref of="TR6BT1Trap14Ctl"() -> (w93:refnum<vi>)
      n45 = control-ref of="TR6BT1Trap15_HCtl"() -> (w90:refnum<vi>)
      n46 = control-ref of="TR6BT1Trap16Ctl"() -> (w89:refnum<vi>)
      n47 = control-ref of="TR6BT1Trap16_HCtl"() -> (w88:refnum<vi>)
      n48 = control-ref of="TR6BT1Trap17Ctl"() -> (w87:refnum<vi>)
      n49 = control-ref of="TR6BT1Trap17_HCtl"() -> (w86:refnum<vi>)
      n50 = control-ref of="TR6BT1Trap18Ctl"() -> (w85:refnum<vi>)
      n51 = control-ref of="TR6BT1Trap18_HCtl"() -> (w84:refnum<vi>)
      n52 = control-ref of="TR6BT1Trap19Ctl"() -> (w83:refnum<vi>)
      n53 = control-ref of="TR6BT1Trap19_HCtl"() -> (w82:refnum<vi>)
      n54 = control-ref of="TR6BT1Trap20Ctl"() -> (w81:refnum<vi>)
      n55 = control-ref of="TR6BT1Trap20_HCtl"() -> (w80:refnum<vi>)
      n56 = control-ref of="TR6BT1Trap21Ctl"() -> (w79:refnum<vi>)
      n57 = control-ref of="TR6BT1Trap21_HCtl"() -> (w78:refnum<vi>)
      n58 = control-ref of="TR6BT1Trap10/2_HCtl"() -> (w58:refnum<vi>)
      n59 = control-ref of="TR6BT1Trap10/2Ctl"() -> (w57:refnum<vi>)
      n60 = control-ref of="TR6BT1Trap11/2_HCtl"() -> (w56:refnum<vi>)
      n61 = control-ref of="TR6BT1Trap11/2Ctl"() -> (w55:refnum<vi>)
      n62 = control-ref of="TR6BT1Trap11/3_HCtl"() -> (w54:refnum<vi>)
      n63 = control-ref of="TR6BT1Trap11/3Ctl"() -> (w53:refnum<vi>)
      n64 = control-ref of="TR6BT1Trap11/4_HCtl"() -> (w52:refnum<vi>)
      n65 = control-ref of="TR6BT1Trap11/4Ctl"() -> (w51:refnum<vi>)
      n66 = control-ref of="TR6BT1Trap11/5_HCtl"() -> (w50:refnum<vi>)
      n67 = control-ref of="TR6BT1Trap11/5Ctl"() -> (w49:refnum<vi>)
      n68 = control-ref of="TR6BT1Trap11/6_HCtl"() -> (w48:refnum<vi>)
      n69 = control-ref of="TR6BT1Trap11/6Ctl"() -> (w47:refnum<vi>)
      n70 = control-ref of="TR6BT1Trap11/7_HCtl"() -> (w46:refnum<vi>)
      n71 = control-ref of="TR6BT1Trap11/7Ctl"() -> (w45:refnum<vi>)
      n72 = control-ref of="TR6BT1Trap11/8_HCtl"() -> (w44:refnum<vi>)
      n73 = control-ref of="TR6BT1Trap11/8Ctl"() -> (w43:refnum<vi>)
      n74 = control-ref of="TR6BT1Trap12/2_HCtl"() -> (w42:refnum<vi>)
      n75 = control-ref of="TR6BT1Trap12/2Ctl"() -> (w41:refnum<vi>)
      n76 = control-ref of="APS_ch1Ctl"() -> (w30:refnum<vi>)
      n77 = control-ref of="APS_ch2Ctl"() -> (w28:refnum<vi>)
      n78 = Build Array(w28, w30, w123, w119, w118, w117, w116, w115, w114, w113, w112, w111, w110, w109, w108, w107, w106, w105, w104, w103, w101, w100, w99, w98, w97, w96, w95, w94, w93, w92, w91, w90, w89, w88, w87, w86, w85, w84, w83, w82, w81, w80, w79, w78, w58, w57, w56, w55, w54, w53, w52, w51, w50, w49, w48, w47, w46, w45, w44, w43, w42, w41) -> (w122:refnum<vi>[])
      n79 = control-ref of="TR6BT1Trap10"() -> (w70:refnum<vi>)
      n80 = control-ref of="TR6BT1Trap13"() -> (w67:refnum<vi>)
      n81 = control-ref of="TR6BT1Trap14"() -> (w66:refnum<vi>)
      n82 = control-ref of="TR6BT1Trap15"() -> (w65:refnum<vi>)
      n83 = control-ref of="TR6BT1Trap19"() -> (w61:refnum<vi>)
      n84 = control-ref of="TR6BT1Trap11"() -> (w69:refnum<vi>)
      n85 = control-ref of="TR6BT1Trap12"() -> (w68:refnum<vi>)
      n86 = control-ref of="TR6BT1Trap17"() -> (w63:refnum<vi>)
      n87 = control-ref of="TR6BT1Trap18"() -> (w62:refnum<vi>)
      n88 = control-ref of="TR6BT1Trap20"() -> (w60:refnum<vi>)
      n89 = control-ref of="TR6BT1Trap21"() -> (w59:refnum<vi>)
      n90 = control-ref of="TR6BT1Trap1"() -> (w121:refnum<vi>)
      n91 = control-ref of="TR6BT1Trap3"() -> (w77:refnum<vi>)
      n92 = control-ref of="TR6BT1Trap4"() -> (w76:refnum<vi>)
      n93 = control-ref of="TR6BT1Trap16"() -> (w64:refnum<vi>)
      n94 = control-ref of="APS_ch1"() -> (w31:refnum<vi>)
      n95 = control-ref of="TR6BT1Trap2"() -> (w102:refnum<vi>)
      n96 = control-ref of="TR6BT1Trap5"() -> (w75:refnum<vi>)
      n97 = control-ref of="TR6BT1Trap6"() -> (w74:refnum<vi>)
      n98 = control-ref of="TR6BT1Trap7"() -> (w73:refnum<vi>)
      n99 = control-ref of="TR6BT1Trap8"() -> (w72:refnum<vi>)
      n100 = control-ref of="TR6BT1Trap9"() -> (w71:refnum<vi>)
      n101 = control-ref of="APS_ch2"() -> (w29:refnum<vi>)
      n102 = control-ref of="TR6BT1Trap11/4"() -> (w37:refnum<vi>)
      n103 = control-ref of="TR6BT1Trap11/5"() -> (w36:refnum<vi>)
      n104 = control-ref of="TR6BT1Trap11/6"() -> (w35:refnum<vi>)
      n105 = control-ref of="TR6BT1Trap11/7"() -> (w34:refnum<vi>)
      n106 = control-ref of="TR6BT1Trap11/8"() -> (w33:refnum<vi>)
      n107 = control-ref of="TR6BT1Trap12/2"() -> (w32:refnum<vi>)
      n108 = control-ref of="TR6BT1Trap10/2"() -> (w40:refnum<vi>)
      n109 = control-ref of="TR6BT1Trap11/2"() -> (w39:refnum<vi>)
      n110 = control-ref of="TR6BT1Trap11/3"() -> (w38:refnum<vi>)
      n111 = Build Array(w29, w31, w121, w102, w77, w76, w75, w74, w73, w72, w71, w70, w69, w68, w67, w66, w65, w64, w63, w62, w61, w60, w59, w40, w39, w38, w37, w36, w35, w34, w33, w32) -> (w120:refnum<vi>[])
      n112 = for {
        tunnel: w122 -> [w129] mode=indexing
        tunnel: w120 -> [w125] mode=indexing
        n113 = call "GUILib.simple numeric init.vi"("ctlRef"=w129, "increment"=1.0) -> ()  [unwired: 16 in, 2 out]
        n114 = call "UtilityLib.set color of boolean.vi"("button"=w125, "valueStatus"=UtilityLib.valueStatus."not implemented", "nOfPair (0)"=1, "setTRUEColor (FALSE)"=TRUE) -> ()  [unwired: 15 in, 1 out]
      }
    }
    frame #2 {
      # "more init"
      n115 = disable-structure shown="Disabled" {
        frame Disabled {
          # "maybe digital stuff...."
          n116 = Build Array() -> (w131:void[])  [unwired: 5 in]
          n117 = Build Array() -> (w130:void[])  [unwired: 5 in]
          n118 = for {
            tunnel: w131 -> [_] mode=indexing
            tunnel: w130 -> [_] mode=indexing
            n119 = call "GUILib.simple boolean init.vi"() -> ()  [unwired: 18 in, 2 out]
            n120 = call "UtilityLib.set color of boolean.vi"("valueStatus"=UtilityLib.valueStatus."not implemented", "nOfPair (0)"=1, "setTRUEColor (FALSE)"=TRUE) -> ()  [unwired: 16 in, 1 out]
          }
        }
        frame Enabled {
        }
      }
    }
    frame #3 {
      # "action"
      n121 = while {
        tunnel: w142 -> [w152]
        tunnel: w141 -> [w150]
        tunnel: w140 -> [w148]
        tunnel: w139 -> [w147]
        tunnel: w138 -> [w146]
        tunnel: w137 -> [w145]
        tunnel: w136 -> [w144]
        tunnel: w135 -> [w143]
        stop <- w149 stop-if-true
        n122 = event shown="[12] \"stop\": Value Change" {
          selector: _ -> [_ _ _ _ _ _ _ _ _ _ _ _ _]
          dyn-events: _ -> [_ _ _ _ _ _ _ _ _ _ _ _ _]
          timeout: -1 -> [_ _ _ _ _ _ _ _ _ _ _ _ _]
          tunnel: w152 -> [_ w157 _ _ w172 _ w178 _ _ _ w442 w447 _]
          tunnel: w150 -> [_ _ _ _ _ _ _ _ _ _ _ _ _]
          tunnel: [_ _ _ _ _ _ _ _ _ _ _ _ "stop"] -> w149
          tunnel: w148 -> [_ w158 _ _ w168 _ _ _ _ _ _ _ _]
          tunnel: w147 -> [_ w154 _ _ _ _ _ _ _ _ _ _ _]
          tunnel: w146 -> [_ w153 _ _ _ _ _ _ _ _ _ _ _]
          tunnel: w145 -> [_ _ _ w165 _ _ w182 _ _ _ _ _ _]
          tunnel: w144 -> [_ _ _ w163 _ _ w176 _ _ _ _ _ _]
          tunnel: w143 -> [_ _ _ _ w167 _ _ _ _ _ _ _ _]
          event Timeout {
            n123 = event-data() -> ()  [unwired: 1 in, 2 out]
          }
          event Value Change {
            n124 = event-data() -> ("NewVal.no link"=w156:bool, "NewVal.data"=w159:string)  [unwired: 1 in]
            n125 = Type Cast(type=T6 [] ("Array"), x=w159) -> (*(type *) &x=w161:T6)
            n126 = Not Equal To 0?(x=w161) -> (x != 0?=w155:bool[])
            n127 = call "GOGControllerGUI.GUI handle ignored controllers.vi"("userEvent"=w157, "controllerNames"=w158, "NOLINK"=w156, "controllersIgnored"=w155, "stateRefs"=w154, "qualityRefs"=w153) -> ()  [unwired: 14 in]
          }
          event Panel Close? {
            n128 = event-data() -> ()  [unwired: 1 in, 4 out]
            n129 = event-data("Discard?"=TRUE) -> ()  [unwired: 1 in, 1 out]
          }
          event "analog1", "TR6BT1Trap1", "TR6BT1Trap2", "TR6BT1Trap3", "TR6BT1Trap4", "TR6BT1Trap5", "TR6BT1Trap6", "TR6BT1Trap7", "TR6BT1Trap8", "TR6BT1Trap9", "TR6BT1Trap10", "TR6BT1Trap11", "TR6BT1Trap12", "TR6BT1Trap13", "TR6BT1Trap14", "TR6BT1Trap15", "TR6BT1Trap16", "TR6BT1Trap17", "TR6BT1Trap18", "TR6BT1Trap19", "TR6BT1Trap20", "TR6BT1Trap21", "TR6BT1Trap10/2", "TR6BT1Trap11/2", "TR6BT1Trap11/3", "TR6BT1Trap11/4", "TR6BT1Trap11/5", "TR6BT1Trap11/6", "TR6BT1Trap11/7", "TR6BT1Trap11/8", "TR6BT1Trap12/2", "TR6BT1 SetMode", "APS_ch1", "APS_ch2": Value Change {
            n130 = event-data() -> ("CtlRef"=w164:refnum<vi>)  [unwired: 1 in]
            n131 = call "GOGControllerGUI.GUI open front panel.vi"("i ref in"=w165, "elementRef"=w164, "controller"=w163) -> ()  [unwired: 15 in, 2 out]
          }
          event "subSystem1", "parentSystem": Value Change {
            n132 = event-data() -> ("CtlRef"=w170:refnum<vi>)  [unwired: 1 in]
            n133 = control-ref of="parentSystem"() -> (w169:refnum<vi>)
            n134 = control-ref of="subSystem1"() -> (w173:refnum<vi>)
            n135 = Build Array (concatenate)(w167, w168) -> (w166:string[])
            n136 = Build Array(w169, w173) -> (w171:refnum<vi>[])
            n137 = call "GOGControllerGUI.GUI set selected subcontroller.vi"("userEvent"=w172, "controllerNames"=w166, "controllerRefs"=w171, "controllerRef"=w170) -> ()  [unwired: 16 in]
          }
          event "TR6BT1Trap1Ctl.inc", "TR6BT1Trap1_HCtl.inc", "TR6BT1Trap2Ctl.inc", "TR6BT1Trap13_HCtl.inc", "TR6BT1Trap13Ctl.inc", "TR6BT1Trap14_HCtl.inc", "TR6BT1Trap14Ctl.inc", "TR6BT1Trap15_HCtl.inc", "TR6BT1Trap16_HCtl.inc", "TR6BT1Trap15Ctl.inc", "TR6BT1Trap16Ctl.inc", "TR6BT1Trap17Ctl.inc", "TR6BT1Trap18Ctl.inc", "TR6BT1Trap19_HCtl.inc", "TR6BT1Trap20Ctl.inc", "TR6BT1Trap18_HCtl.inc", "TR6BT1Trap17_HCtl.inc", "TR6BT1Trap20_HCtl.inc", "TR6BT1Trap19Ctl.inc", "TR6BT1Trap3_HCtl.inc", "TR6BT1Trap3Ctl.inc", "TR6BT1Trap5_HCtl.inc", "TR6BT1Trap6_HCtl.inc", "TR6BT1Trap6Ctl.inc", "TR6BT1Trap8Ctl.inc", "TR6BT1Trap21Ctl.inc", "TR6BT1Trap12Ctl.inc", "TR6BT1Trap5Ctl.inc", "TR6BT1Trap7Ctl.inc", "TR6BT1Trap7_HCtl.inc", "TR6BT1Trap8_HCtl.inc", "TR6BT1Trap21_HCtl.inc", "TR6BT1Trap12_HCtl.inc", "TR6BT1Trap9_HCtl.inc", "TR6BT1Trap4_HCtl.inc", "TR6BT1Trap9Ctl.inc", "TR6BT1Trap10_HCtl.inc", "TR6BT1Trap10Ctl.inc", "TR6BT1Trap11Ctl.inc", "TR6BT1Trap11_HCtl.inc": Value Change {
            n138 = event-data() -> ("CtlRef"=w175:refnum<vi>, "NewVal"=w174:dbl)  [unwired: 1 in]
            n139 = call "GUILib.simple numeric change increment.vi"("ctlRef"=w175, "increment"=w174) -> ()  [unwired: 16 in, 2 out]
          }
          event Value Change {
            n140 = event-data() -> ("CtlRef"=w181:refnum<vi>, "NewVal"=w180:T3)  [unwired: 1 in]
            n141 = call-poly "CoreLib.data 2 byte array.vi"("f64"=w180) -> ("byteArray out"=w179:T6)  [unwired: 18 in]
            n142 = call "GOGControllerGUI.GUI set nominal value.vi"("i ref in"=w182, "nominalRef"=w181, "nominalData"=w179, "controller"=w176) -> ("error out"=w177:errorcluster)  [unwired: 14 in, 1 out]
            n143 = call "GOGControllerGUI.GUI set error.vi"("userEvent"=w178, "controller"=w176, "GUIError"=w177) -> ()  [unwired: 16 in, 1 out]
          }
          event "LowVoltage      HighVoltage": Value Change {
            n144 = event-data() -> ()  [unwired: 1 in, 6 out]
            n145 = property on="TR6BT1Trap1_HCtl" class="Clust (strict)"("Visible"="LowVoltage      HighVoltage") -> ()  [unwired: 2 in, 2 out]
            n146 = property on="TR6BT1Trap2_HCtl" class="Clust (strict)"("Visible"="LowVoltage      HighVoltage") -> ()  [unwired: 2 in, 2 out]
            n147 = property on="TR6BT1Trap3_HCtl" class="Clust (strict)"("Visible"="LowVoltage      HighVoltage") -> ()  [unwired: 2 in, 2 out]
            n148 = property on="TR6BT1Trap4_HCtl" class="Clust (strict)"("Visible"="LowVoltage      HighVoltage") -> ()  [unwired: 2 in, 2 out]
            n149 = property on="TR6BT1Trap5_HCtl" class="Clust (strict)"("Visible"="LowVoltage      HighVoltage") -> ()  [unwired: 2 in, 2 out]
            n150 = property on="TR6BT1Trap6_HCtl" class="Clust (strict)"("Visible"="LowVoltage      HighVoltage") -> ()  [unwired: 2 in, 2 out]
            n151 = property on="TR6BT1Trap7_HCtl" class="Clust (strict)"("Visible"="LowVoltage      HighVoltage") -> ()  [unwired: 2 in, 2 out]
            n152 = property on="TR6BT1Trap8_HCtl" class="Clust (strict)"("Visible"="LowVoltage      HighVoltage") -> ()  [unwired: 2 in, 2 out]
            n153 = property on="TR6BT1Trap9_HCtl" class="Clust (strict)"("Visible"="LowVoltage      HighVoltage") -> ()  [unwired: 2 in, 2 out]
            n154 = property on="TR6BT1Trap10_HCtl" class="Clust (strict)"("Visible"="LowVoltage      HighVoltage") -> ()  [unwired: 2 in, 2 out]
            n155 = property on="TR6BT1Trap12_HCtl" class="Clust (strict)"("Visible"="LowVoltage      HighVoltage") -> ()  [unwired: 2 in, 2 out]
            n156 = property on="TR6BT1Trap13_HCtl" class="Clust (strict)"("Visible"="LowVoltage      HighVoltage") -> ()  [unwired: 2 in, 2 out]
            n157 = property on="TR6BT1Trap11_HCtl" class="Clust (strict)"("Visible"="LowVoltage      HighVoltage") -> ()  [unwired: 2 in, 2 out]
            n158 = Not(x="LowVoltage      HighVoltage") -> (.not. x?=w185:bool)
            n159 = property on="TR6BT1Trap14_HCtl" class="Clust (strict)"("Visible"="LowVoltage      HighVoltage") -> ()  [unwired: 2 in, 2 out]
            n160 = property on="TR6BT1Trap15_HCtl" class="Clust (strict)"("Visible"="LowVoltage      HighVoltage") -> ()  [unwired: 2 in, 2 out]
            n161 = property on="TR6BT1Trap16_HCtl" class="Clust (strict)"("Visible"="LowVoltage      HighVoltage") -> ()  [unwired: 2 in, 2 out]
            n162 = property on="TR6BT1Trap17_HCtl" class="Clust (strict)"("Visible"="LowVoltage      HighVoltage") -> ()  [unwired: 2 in, 2 out]
            n163 = property on="TR6BT1Trap18_HCtl" class="Clust (strict)"("Visible"="LowVoltage      HighVoltage") -> ()  [unwired: 2 in, 2 out]
            n164 = property on="TR6BT1Trap19_HCtl" class="Clust (strict)"("Visible"="LowVoltage      HighVoltage") -> ()  [unwired: 2 in, 2 out]
            n165 = property on="TR6BT1Trap20_HCtl" class="Clust (strict)"("Visible"="LowVoltage      HighVoltage") -> ()  [unwired: 2 in, 2 out]
            n166 = property on="TR6BT1Trap21_HCtl" class="Clust (strict)"("Visible"="LowVoltage      HighVoltage") -> ()  [unwired: 2 in, 2 out]
            n167 = property on="TR6BT1Trap1Ctl" class="Clust (strict)"("Visible"=w185) -> ()  [unwired: 2 in, 2 out]
            n168 = property on="TR6BT1Trap2Ctl" class="Clust (strict)"("Visible"=w185) -> ()  [unwired: 2 in, 2 out]
            n169 = property on="TR6BT1Trap3Ctl" class="Clust (strict)"("Visible"=w185) -> ()  [unwired: 2 in, 2 out]
            n170 = property on="TR6BT1Trap4Ctl" class="Clust (strict)"("Visible"=w185) -> ()  [unwired: 2 in, 2 out]
            n171 = property on="TR6BT1Trap5Ctl" class="Clust (strict)"("Visible"=w185) -> ()  [unwired: 2 in, 2 out]
            n172 = property on="TR6BT1Trap6Ctl" class="Clust (strict)"("Visible"=w185) -> ()  [unwired: 2 in, 2 out]
            n173 = property on="TR6BT1Trap8Ctl" class="Clust (strict)"("Visible"=w185) -> ()  [unwired: 2 in, 2 out]
            n174 = property on="TR6BT1Trap9Ctl" class="Clust (strict)"("Visible"=w185) -> ()  [unwired: 2 in, 2 out]
            n175 = property on="TR6BT1Trap10Ctl" class="Clust (strict)"("Visible"=w185) -> ()  [unwired: 2 in, 2 out]
            n176 = property on="TR6BT1Trap11Ctl" class="Clust (strict)"("Visible"=w185) -> ()  [unwired: 2 in, 2 out]
            n177 = property on="TR6BT1Trap12Ctl" class="Clust (strict)"("Visible"=w185) -> ()  [unwired: 2 in, 2 out]
            n178 = property on="TR6BT1Trap13Ctl" class="Clust (strict)"("Visible"=w185) -> ()  [unwired: 2 in, 2 out]
            n179 = property on="TR6BT1Trap14Ctl" class="Clust (strict)"("Visible"=w185) -> ()  [unwired: 2 in, 2 out]
            n180 = property on="TR6BT1Trap15Ctl" class="Clust (strict)"("Visible"=w185) -> ()  [unwired: 2 in, 2 out]
            n181 = property on="TR6BT1Trap16Ctl" class="Clust (strict)"("Visible"=w185) -> ()  [unwired: 2 in, 2 out]
            n182 = property on="TR6BT1Trap17Ctl" class="Clust (strict)"("Visible"=w185) -> ()  [unwired: 2 in, 2 out]
            n183 = property on="TR6BT1Trap18Ctl" class="Clust (strict)"("Visible"=w185) -> ()  [unwired: 2 in, 2 out]
            n184 = property on="TR6BT1Trap19Ctl" class="Clust (strict)"("Visible"=w185) -> ()  [unwired: 2 in, 2 out]
            n185 = property on="TR6BT1Trap20Ctl" class="Clust (strict)"("Visible"=w185) -> ()  [unwired: 2 in, 2 out]
            n186 = property on="TR6BT1Trap21Ctl" class="Clust (strict)"("Visible"=w185) -> ()  [unwired: 2 in, 2 out]
            n187 = property on="TR6BT1Trap7Ctl" class="Clust (strict)"("Visible"=w185) -> ()  [unwired: 2 in, 2 out]
            n188 = case shown="\"Voltage2\"" "Enum" {
              frame "Voltage1", Default {
              }
              frame "Voltage2" {
              }
            }
          }
          event "High1", "High2", "High3", "High4", "High5", "High6", "High7", "High8", "High9", "High10", "High11", "High12", "High13", "High14", "High15", "High16", "High17", "High18", "High19", "High20", "High21": Value Change {
            n189 = event-data() -> ()  [unwired: 1 in, 6 out]
            n190 = property on="nom" class="DigNum (strict)"() -> ("Value"=w295:T3)  [unwired: 2 in, 2 out]
            n191 = property on="nom" class="DigNum (strict)"() -> ("Value"=w294:T3)  [unwired: 2 in, 2 out]
            n192 = property on="nom" class="DigNum (strict)"() -> ("Value"=w293:T3)  [unwired: 2 in, 2 out]
            n193 = property on="nom" class="DigNum (strict)"() -> ("Value"=w292:T3)  [unwired: 2 in, 2 out]
            n194 = property on="nom" class="DigNum (strict)"() -> ("Value"=w291:T3)  [unwired: 2 in, 2 out]
            n195 = property on="nom" class="DigNum (strict)"() -> ("Value"=w290:T3)  [unwired: 2 in, 2 out]
            n196 = property on="nom" class="DigNum (strict)"() -> ("Value"=w289:T3)  [unwired: 2 in, 2 out]
            n197 = property on="nom" class="DigNum (strict)"() -> ("Value"=w288:T3)  [unwired: 2 in, 2 out]
            n198 = property on="nom" class="DigNum (strict)"() -> ("Value"=w275:T3)  [unwired: 2 in, 2 out]
            n199 = property on="nom" class="DigNum (strict)"() -> ("Value"=w274:T3)  [unwired: 2 in, 2 out]
            n200 = property on="nom" class="DigNum (strict)"() -> ("Value"=w273:T3)  [unwired: 2 in, 2 out]
            n201 = property on="nom" class="DigNum (strict)"() -> ("Value"=w272:T3)  [unwired: 2 in, 2 out]
            n202 = property on="nom" class="DigNum (strict)"() -> ("Value"=w271:T3)  [unwired: 2 in, 2 out]
            n203 = property on="nom" class="DigNum (strict)"() -> ("Value"=w270:T3)  [unwired: 2 in, 2 out]
            n204 = property on="nom" class="DigNum (strict)"() -> ("Value"=w269:T3)  [unwired: 2 in, 2 out]
            n205 = property on="nom" class="DigNum (strict)"() -> ("Value"=w268:T3)  [unwired: 2 in, 2 out]
            n206 = Select(t=w295, s="High1", f=w294) -> (s? t:f=w305:T3)
            n207 = Select(t=w293, s="High2", f=w292) -> (s? t:f=w302:T3)
            n208 = Select(t=w291, s="High3", f=w290) -> (s? t:f=w301:T3)
            n209 = Select(t=w289, s="High4", f=w288) -> (s? t:f=w300:T3)
            n210 = Select(t=w275, s="High5", f=w274) -> (s? t:f=w280:T3)
            n211 = Select(t=w273, s="High6", f=w272) -> (s? t:f=w283:T3)
            n212 = Select(t=w271, s="High7", f=w270) -> (s? t:f=w284:T3)
            n213 = Select(t=w269, s="High8", f=w268) -> (s? t:f=w285:T3)
            n214 = Bundle(0.5, "Value"=w305) -> (w310:cluster{dbl, "Value":T3})  [unwired: 1 in]
            n215 = Bundle(1.5, "Value"=w302) -> (w311:cluster{dbl, "Value":T3})  [unwired: 1 in]
            n216 = Bundle(2.5, "Value"=w301) -> (w297:cluster{dbl, "Value":T3})  [unwired: 1 in]
            n217 = Bundle(3.5, "Value"=w300) -> (w296:cluster{dbl, "Value":T3})  [unwired: 1 in]
            n218 = Bundle(4.5, "Value"=w280) -> (w267:cluster{dbl, "Value":T3})  [unwired: 1 in]
            n219 = Bundle(5.5, "Value"=w283) -> (w266:cluster{dbl, "Value":T3})  [unwired: 1 in]
            n220 = Bundle(6.5, "Value"=w284) -> (w265:cluster{dbl, "Value":T3})  [unwired: 1 in]
            n221 = Bundle(7.5, "Value"=w285) -> (w264:cluster{dbl, "Value":T3})  [unwired: 1 in]
            n222 = property on="nom" class="DigNum (strict)"() -> ("Value"=w239:T3)  [unwired: 2 in, 2 out]
            n223 = property on="nom" class="DigNum (strict)"() -> ("Value"=w238:T3)  [unwired: 2 in, 2 out]
            n224 = property on="nom" class="DigNum (strict)"() -> ("Value"=w237:T3)  [unwired: 2 in, 2 out]
            n225 = property on="nom" class="DigNum (strict)"() -> ("Value"=w236:T3)  [unwired: 2 in, 2 out]
            n226 = property on="nom" class="DigNum (strict)"() -> ("Value"=w235:T3)  [unwired: 2 in, 2 out]
            n227 = property on="nom" class="DigNum (strict)"() -> ("Value"=w234:T3)  [unwired: 2 in, 2 out]
            n228 = property on="nom" class="DigNum (strict)"() -> ("Value"=w233:T3)  [unwired: 2 in, 2 out]
            n229 = property on="nom" class="DigNum (strict)"() -> ("Value"=w232:T3)  [unwired: 2 in, 2 out]
            n230 = property on="nom" class="DigNum (strict)"() -> ("Value"=w231:T3)  [unwired: 2 in, 2 out]
            n231 = property on="nom" class="DigNum (strict)"() -> ("Value"=w230:T3)  [unwired: 2 in, 2 out]
            n232 = property on="nom" class="DigNum (strict)"() -> ("Value"=w229:T3)  [unwired: 2 in, 2 out]
            n233 = property on="nom" class="DigNum (strict)"() -> ("Value"=w228:T3)  [unwired: 2 in, 2 out]
            n234 = property on="nom" class="DigNum (strict)"() -> ("Value"=w227:T3)  [unwired: 2 in, 2 out]
            n235 = property on="nom" class="DigNum (strict)"() -> ("Value"=w226:T3)  [unwired: 2 in, 2 out]
            n236 = Select(t=w239, s="High9", f=w238) -> (s? t:f=w261:T3)
            n237 = Select(t=w237, s="High10", f=w236) -> (s? t:f=w260:T3)
            n238 = Select(t=w235, s="High11", f=w234) -> (s? t:f=w254:T3)
            n239 = Select(t=w233, s="High12", f=w232) -> (s? t:f=w255:T3)
            n240 = Select(t=w231, s="High13", f=w230) -> (s? t:f=w249:T3)
            n241 = Select(t=w229, s="High14", f=w228) -> (s? t:f=w248:T3)
            n242 = Select(t=w227, s="High15", f=w226) -> (s? t:f=w242:T3)
            n243 = Bundle(8.5, "Value"=w261) -> (w225:cluster{dbl, "Value":T3})  [unwired: 1 in]
            n244 = Bundle(9.5, "Value"=w260) -> (w224:cluster{dbl, "Value":T3})  [unwired: 1 in]
            n245 = Bundle(10.5, "Value"=w254) -> (w223:cluster{dbl, "Value":T3})  [unwired: 1 in]
            n246 = Bundle(11.5, "Value"=w255) -> (w222:cluster{dbl, "Value":T3})  [unwired: 1 in]
            n247 = Bundle(12.5, "Value"=w249) -> (w221:cluster{dbl, "Value":T3})  [unwired: 1 in]
            n248 = Bundle(13.5, "Value"=w248) -> (w220:cluster{dbl, "Value":T3})  [unwired: 1 in]
            n249 = Bundle(14.5, "Value"=w242) -> (w219:cluster{dbl, "Value":T3})  [unwired: 1 in]
            n250 = property on="nom" class="DigNum (strict)"() -> ("Value"=w203:T3)  [unwired: 2 in, 2 out]
            n251 = property on="nom" class="DigNum (strict)"() -> ("Value"=w202:T3)  [unwired: 2 in, 2 out]
            n252 = property on="nom" class="DigNum (strict)"() -> ("Value"=w201:T3)  [unwired: 2 in, 2 out]
            n253 = property on="nom" class="DigNum (strict)"() -> ("Value"=w200:T3)  [unwired: 2 in, 2 out]
            n254 = property on="nom" class="DigNum (strict)"() -> ("Value"=w199:T3)  [unwired: 2 in, 2 out]
            n255 = property on="nom" class="DigNum (strict)"() -> ("Value"=w198:T3)  [unwired: 2 in, 2 out]
            n256 = property on="nom" class="DigNum (strict)"() -> ("Value"=w197:T3)  [unwired: 2 in, 2 out]
            n257 = property on="nom" class="DigNum (strict)"() -> ("Value"=w196:T3)  [unwired: 2 in, 2 out]
            n258 = property on="nom" class="DigNum (strict)"() -> ("Value"=w195:T3)  [unwired: 2 in, 2 out]
            n259 = property on="nom" class="DigNum (strict)"() -> ("Value"=w194:T3)  [unwired: 2 in, 2 out]
            n260 = property on="nom" class="DigNum (strict)"() -> ("Value"=w193:T3)  [unwired: 2 in, 2 out]
            n261 = property on="nom" class="DigNum (strict)"() -> ("Value"=w192:T3)  [unwired: 2 in, 2 out]
            n262 = Select(t=w203, s="High16", f=w202) -> (s? t:f=w243:T3)
            n263 = Select(t=w195, s="High20", f=w194) -> (s? t:f=w208:T3)
            n264 = Select(t=w199, s="High18", f=w198) -> (s? t:f=w214:T3)
            n265 = Select(t=w197, s="High19", f=w196) -> (s? t:f=w211:T3)
            n266 = Select(t=w201, s="High17", f=w200) -> (s? t:f=w217:T3)
            n267 = Select(t=w193, s="High21", f=w192) -> (s? t:f=w205:T3)
            n268 = Bundle(15.5, "Value"=w243) -> (w191:cluster{dbl, "Value":T3})  [unwired: 1 in]
            n269 = Bundle(18.5, "Value"=w211) -> (w188:cluster{dbl, "Value":T3})  [unwired: 1 in]
            n270 = Bundle(17.5, "Value"=w214) -> (w189:cluster{dbl, "Value":T3})  [unwired: 1 in]
            n271 = Bundle(19.5, "Value"=w208) -> (w187:cluster{dbl, "Value":T3})  [unwired: 1 in]
            n272 = Bundle(16.5, "Value"=w217) -> (w190:cluster{dbl, "Value":T3})  [unwired: 1 in]
            n273 = Bundle(20.5, "Value"=w205) -> (w186:cluster{dbl, "Value":T3})  [unwired: 1 in]
            n274 = Build Array(w310, w311, w297, w296, w267, w266, w265, w264, w225, w224, w223, w222, w221, w220, w219, w191, w190, w189, w188, w187, w186) -> (→"XY Graph":cluster{dbl, "Value":T3}[])
          }
          event "All Low   All High": Value Change {
            n275 = event-data() -> ()  [unwired: 1 in, 6 out]
            n276 = case shown="False" "All Low   All High" {
              frame True {
                n277 = property on="nom" class="DigNum (strict)"() -> ("Value"=w335:T3)  [unwired: 2 in, 2 out]
                n278 = property on="nom" class="DigNum (strict)"() -> ("Value"=w334:T3)  [unwired: 2 in, 2 out]
                n279 = property on="nom" class="DigNum (strict)"() -> ("Value"=w333:T3)  [unwired: 2 in, 2 out]
                n280 = property on="nom" class="DigNum (strict)"() -> ("Value"=w332:T3)  [unwired: 2 in, 2 out]
                n281 = property on="nom" class="DigNum (strict)"() -> ("Value"=w331:T3)  [unwired: 2 in, 2 out]
                n282 = property on="nom" class="DigNum (strict)"() -> ("Value"=w330:T3)  [unwired: 2 in, 2 out]
                n283 = property on="nom" class="DigNum (strict)"() -> ("Value"=w329:T3)  [unwired: 2 in, 2 out]
                n284 = property on="nom" class="DigNum (strict)"() -> ("Value"=w328:T3)  [unwired: 2 in, 2 out]
                n285 = property on="nom" class="DigNum (strict)"() -> ("Value"=w327:T3)  [unwired: 2 in, 2 out]
                n286 = property on="nom" class="DigNum (strict)"() -> ("Value"=w326:T3)  [unwired: 2 in, 2 out]
                n287 = property on="nom" class="DigNum (strict)"() -> ("Value"=w325:T3)  [unwired: 2 in, 2 out]
                n288 = property on="nom" class="DigNum (strict)"() -> ("Value"=w324:T3)  [unwired: 2 in, 2 out]
                n289 = property on="nom" class="DigNum (strict)"() -> ("Value"=w323:T3)  [unwired: 2 in, 2 out]
                n290 = property on="nom" class="DigNum (strict)"() -> ("Value"=w322:T3)  [unwired: 2 in, 2 out]
                n291 = property on="nom" class="DigNum (strict)"() -> ("Value"=w321:T3)  [unwired: 2 in, 2 out]
                n292 = Bundle(0.5, "Value"=w335) -> (w337:cluster{dbl, "Value":T3})  [unwired: 1 in]
                n293 = Bundle(1.5, "Value"=w334) -> (w336:cluster{dbl, "Value":T3})  [unwired: 1 in]
                n294 = Bundle(2.5, "Value"=w333) -> (w342:cluster{dbl, "Value":T3})  [unwired: 1 in]
                n295 = Bundle(3.5, "Value"=w332) -> (w343:cluster{dbl, "Value":T3})  [unwired: 1 in]
                n296 = Bundle(4.5, "Value"=w331) -> (w348:cluster{dbl, "Value":T3})  [unwired: 1 in]
                n297 = Bundle(5.5, "Value"=w330) -> (w349:cluster{dbl, "Value":T3})  [unwired: 1 in]
                n298 = Bundle(6.5, "Value"=w329) -> (w350:cluster{dbl, "Value":T3})  [unwired: 1 in]
                n299 = Bundle(9.5, "Value"=w326) -> (w361:cluster{dbl, "Value":T3})  [unwired: 1 in]
                n300 = Bundle(8.5, "Value"=w327) -> (w360:cluster{dbl, "Value":T3})  [unwired: 1 in]
                n301 = Bundle(7.5, "Value"=w328) -> (w351:cluster{dbl, "Value":T3})  [unwired: 1 in]
                n302 = Bundle(10.5, "Value"=w325) -> (w362:cluster{dbl, "Value":T3})  [unwired: 1 in]
                n303 = Bundle(11.5, "Value"=w324) -> (w363:cluster{dbl, "Value":T3})  [unwired: 1 in]
                n304 = Bundle(12.5, "Value"=w323) -> (w364:cluster{dbl, "Value":T3})  [unwired: 1 in]
                n305 = Bundle(13.5, "Value"=w322) -> (w365:cluster{dbl, "Value":T3})  [unwired: 1 in]
                n306 = Bundle(14.5, "Value"=w321) -> (w366:cluster{dbl, "Value":T3})  [unwired: 1 in]
                n307 = property on="nom" class="DigNum (strict)"() -> ("Value"=w320:T3)  [unwired: 2 in, 2 out]
                n308 = property on="nom" class="DigNum (strict)"() -> ("Value"=w319:T3)  [unwired: 2 in, 2 out]
                n309 = property on="nom" class="DigNum (strict)"() -> ("Value"=w318:T3)  [unwired: 2 in, 2 out]
                n310 = property on="nom" class="DigNum (strict)"() -> ("Value"=w317:T3)  [unwired: 2 in, 2 out]
                n311 = property on="nom" class="DigNum (strict)"() -> ("Value"=w316:T3)  [unwired: 2 in, 2 out]
                n312 = property on="nom" class="DigNum (strict)"() -> ("Value"=w315:T3)  [unwired: 2 in, 2 out]
                n313 = Bundle(15.5, "Value"=w320) -> (w372:cluster{dbl, "Value":T3})  [unwired: 1 in]
                n314 = Bundle(16.5, "Value"=w319) -> (w373:cluster{dbl, "Value":T3})  [unwired: 1 in]
                n315 = Bundle(17.5, "Value"=w318) -> (w374:cluster{dbl, "Value":T3})  [unwired: 1 in]
                n316 = Bundle(18.5, "Value"=w317) -> (w375:cluster{dbl, "Value":T3})  [unwired: 1 in]
                n317 = Bundle(19.5, "Value"=w316) -> (w376:cluster{dbl, "Value":T3})  [unwired: 1 in]
                n318 = Bundle(20.5, "Value"=w315) -> (w377:cluster{dbl, "Value":T3})  [unwired: 1 in]
                n319 = Build Array(w337, w336, w342, w343, w348, w349, w350, w351, w360, w361, w362, w363, w364, w365, w366, w372, w373, w374, w375, w376, w377) -> (w314:cluster{dbl, "Value":T3}[])
                n320 = property on="XY Graph" class="XYGraph (strict)"("Value"=w314) -> ()  [unwired: 2 in, 2 out]
              }
              frame False {
                n321 = property on="nom" class="DigNum (strict)"() -> ("Value"=w400:T3)  [unwired: 2 in, 2 out]
                n322 = property on="nom" class="DigNum (strict)"() -> ("Value"=w399:T3)  [unwired: 2 in, 2 out]
                n323 = property on="nom" class="DigNum (strict)"() -> ("Value"=w398:T3)  [unwired: 2 in, 2 out]
                n324 = property on="nom" class="DigNum (strict)"() -> ("Value"=w397:T3)  [unwired: 2 in, 2 out]
                n325 = property on="nom" class="DigNum (strict)"() -> ("Value"=w396:T3)  [unwired: 2 in, 2 out]
                n326 = property on="nom" class="DigNum (strict)"() -> ("Value"=w395:T3)  [unwired: 2 in, 2 out]
                n327 = property on="nom" class="DigNum (strict)"() -> ("Value"=w394:T3)  [unwired: 2 in, 2 out]
                n328 = property on="nom" class="DigNum (strict)"() -> ("Value"=w393:T3)  [unwired: 2 in, 2 out]
                n329 = property on="nom" class="DigNum (strict)"() -> ("Value"=w392:T3)  [unwired: 2 in, 2 out]
                n330 = property on="nom" class="DigNum (strict)"() -> ("Value"=w391:T3)  [unwired: 2 in, 2 out]
                n331 = property on="nom" class="DigNum (strict)"() -> ("Value"=w390:T3)  [unwired: 2 in, 2 out]
                n332 = property on="nom" class="DigNum (strict)"() -> ("Value"=w389:T3)  [unwired: 2 in, 2 out]
                n333 = property on="nom" class="DigNum (strict)"() -> ("Value"=w388:T3)  [unwired: 2 in, 2 out]
                n334 = Bundle(8.5, "Value"=w392) -> (w425:cluster{dbl, "Value":T3})  [unwired: 1 in]
                n335 = Bundle(9.5, "Value"=w391) -> (w426:cluster{dbl, "Value":T3})  [unwired: 1 in]
                n336 = Bundle(10.5, "Value"=w390) -> (w427:cluster{dbl, "Value":T3})  [unwired: 1 in]
                n337 = Bundle(11.5, "Value"=w389) -> (w379:cluster{dbl, "Value":T3})  [unwired: 1 in]
                n338 = Bundle(12.5, "Value"=w388) -> (w428:cluster{dbl, "Value":T3})  [unwired: 1 in]
                n339 = Bundle(0.5, "Value"=w400) -> (w402:cluster{dbl, "Value":T3})  [unwired: 1 in]
                n340 = Bundle(1.5, "Value"=w399) -> (w401:cluster{dbl, "Value":T3})  [unwired: 1 in]
                n341 = Bundle(2.5, "Value"=w398) -> (w407:cluster{dbl, "Value":T3})  [unwired: 1 in]
                n342 = Bundle(3.5, "Value"=w397) -> (w408:cluster{dbl, "Value":T3})  [unwired: 1 in]
                n343 = Bundle(4.5, "Value"=w396) -> (w413:cluster{dbl, "Value":T3})  [unwired: 1 in]
                n344 = Bundle(5.5, "Value"=w395) -> (w414:cluster{dbl, "Value":T3})  [unwired: 1 in]
                n345 = Bundle(6.5, "Value"=w394) -> (w415:cluster{dbl, "Value":T3})  [unwired: 1 in]
                n346 = Bundle(7.5, "Value"=w393) -> (w416:cluster{dbl, "Value":T3})  [unwired: 1 in]
                n347 = property on="nom" class="DigNum (strict)"() -> ("Value"=w387:T3)  [unwired: 2 in, 2 out]
                n348 = property on="nom" class="DigNum (strict)"() -> ("Value"=w386:T3)  [unwired: 2 in, 2 out]
                n349 = property on="nom" class="DigNum (strict)"() -> ("Value"=w385:T3)  [unwired: 2 in, 2 out]
                n350 = property on="nom" class="DigNum (strict)"() -> ("Value"=w384:T3)  [unwired: 2 in, 2 out]
                n351 = property on="nom" class="DigNum (strict)"() -> ("Value"=w383:T3)  [unwired: 2 in, 2 out]
                n352 = property on="nom" class="DigNum (strict)"() -> ("Value"=w382:T3)  [unwired: 2 in, 2 out]
                n353 = property on="nom" class="DigNum (strict)"() -> ("Value"=w381:T3)  [unwired: 2 in, 2 out]
                n354 = property on="nom" class="DigNum (strict)"() -> ("Value"=w380:T3)  [unwired: 2 in, 2 out]
                n355 = Bundle(13.5, "Value"=w387) -> (w429:cluster{dbl, "Value":T3})  [unwired: 1 in]
                n356 = Bundle(14.5, "Value"=w386) -> (w430:cluster{dbl, "Value":T3})  [unwired: 1 in]
                n357 = Bundle(15.5, "Value"=w385) -> (w436:cluster{dbl, "Value":T3})  [unwired: 1 in]
                n358 = Bundle(16.5, "Value"=w384) -> (w437:cluster{dbl, "Value":T3})  [unwired: 1 in]
                n359 = Bundle(17.5, "Value"=w383) -> (w438:cluster{dbl, "Value":T3})  [unwired: 1 in]
                n360 = Bundle(18.5, "Value"=w382) -> (w439:cluster{dbl, "Value":T3})  [unwired: 1 in]
                n361 = Bundle(20.5, "Value"=w380) -> (w441:cluster{dbl, "Value":T3})  [unwired: 1 in]
                n362 = Bundle(19.5, "Value"=w381) -> (w440:cluster{dbl, "Value":T3})  [unwired: 1 in]
                n363 = Build Array(w402, w401, w407, w408, w413, w414, w415, w416, w425, w426, w427, w379, w428, w429, w430, w436, w437, w438, w439, w440, w441) -> (w378:cluster{dbl, "Value":T3}[])
                n364 = property on="XY Graph" class="XYGraph (strict)"("Value"=w378) -> ()  [unwired: 2 in, 2 out]
              }
            }
            n365 = property on="High1" class="Bool (strict)"("Value"="All Low   All High") -> ()  [unwired: 2 in, 2 out]
            n366 = property on="High2" class="Bool (strict)"("Value"="All Low   All High") -> ()  [unwired: 2 in, 2 out]
            n367 = property on="High3" class="Bool (strict)"("Value"="All Low   All High") -> ()  [unwired: 2 in, 2 out]
            n368 = property on="High4" class="Bool (strict)"("Value"="All Low   All High") -> ()  [unwired: 2 in, 2 out]
            n369 = property on="High5" class="Bool (strict)"("Value"="All Low   All High") -> ()  [unwired: 2 in, 2 out]
            n370 = property on="High6" class="Bool (strict)"("Value"="All Low   All High") -> ()  [unwired: 2 in, 2 out]
            n371 = property on="High7" class="Bool (strict)"("Value"="All Low   All High") -> ()  [unwired: 2 in, 2 out]
            n372 = property on="High8" class="Bool (strict)"("Value"="All Low   All High") -> ()  [unwired: 2 in, 2 out]
            n373 = property on="High9" class="Bool (strict)"("Value"="All Low   All High") -> ()  [unwired: 2 in, 2 out]
            n374 = property on="High10" class="Bool (strict)"("Value"="All Low   All High") -> ()  [unwired: 2 in, 2 out]
            n375 = property on="High11" class="Bool (strict)"("Value"="All Low   All High") -> ()  [unwired: 2 in, 2 out]
            n376 = property on="High12" class="Bool (strict)"("Value"="All Low   All High") -> ()  [unwired: 2 in, 2 out]
            n377 = property on="High13" class="Bool (strict)"("Value"="All Low   All High") -> ()  [unwired: 2 in, 2 out]
            n378 = property on="High14" class="Bool (strict)"("Value"="All Low   All High") -> ()  [unwired: 2 in, 2 out]
            n379 = property on="High15" class="Bool (strict)"("Value"="All Low   All High") -> ()  [unwired: 2 in, 2 out]
            n380 = property on="High16" class="Bool (strict)"("Value"="All Low   All High") -> ()  [unwired: 2 in, 2 out]
            n381 = property on="High17" class="Bool (strict)"("Value"="All Low   All High") -> ()  [unwired: 2 in, 2 out]
            n382 = property on="High18" class="Bool (strict)"("Value"="All Low   All High") -> ()  [unwired: 2 in, 2 out]
            n383 = property on="High19" class="Bool (strict)"("Value"="All Low   All High") -> ()  [unwired: 2 in, 2 out]
            n384 = property on="High20" class="Bool (strict)"("Value"="All Low   All High") -> ()  [unwired: 2 in, 2 out]
            n385 = property on="High21" class="Bool (strict)"("Value"="All Low   All High") -> ()  [unwired: 2 in, 2 out]
          }
          event "Previous": Value Change {
            n386 = event-data() -> ()  [unwired: 1 in, 6 out]
            n387 = Bundle By Name(cluster="userEventsMain", "data"="HTLE_TR5", "dataType"=0) -> (w446:T1)
            n388 = Generate User Event(user event=w442, event data cluster=w446) -> ()  [unwired: 2 in, 2 out]
          }
          event "Next": Value Change {
            n389 = event-data() -> ()  [unwired: 1 in, 6 out]
            n390 = Bundle By Name(cluster="userEventsMain 2", "data"="HTLE_TR6-LowerPart", "dataType"=0) -> (w451:T1)
            n391 = Generate User Event(user event=w447, event data cluster=w451) -> ()  [unwired: 2 in, 2 out]
          }
          event "stop": Value Change {
            n392 = event-data() -> ()  [unwired: 1 in, 6 out]
          }
        }
      }
    }
    frame #4 {
      # "deinit"
      n393 = call "DimIndicators.dic_release_service.vi"("controlRef"=w453) -> ()  [unwired: 18 in, 1 out]
    }
  }
